vi "Manual splitting analysis.vi"() -> ()   [LabVIEW 2013]
uses:
  <vilib>/Math Plots/2D Math Plots/2D Error Bar/2D Error Bar XCtrl/2D Error Bar.xctl
  <vilib>/Math Plots/2D Math Plots/2D Error Bar/2D Error Bar Datatype/2D Error Bar Datatype.lvclass
  <vilib>/Math Plots/2D Math Plots/2D Error Bar/2D Error Bar Datatype/Public/Plot Helper (Percentage).vi
  <vilib>/Analysis/NI_AALPro.lvlib
panel:
  out "Tab Control":enum32{"Page 1", "Page 2", "ITX"}(tab)=enum."ITX"
  in  "OK Button":bool
  in  "Peak Detector":cluster{"X":dbl, "Y":dbl}[](graph)=[{"X"=-0.049280000000000004, "Y"=-90000.0}, {"X"=-0.04744, "Y"=-90000.0}, {"X"=-0.044360000000000004, "Y"=-90000.0}, {"X"=-0.04356, "Y"=-90000.0}, {"X"=-0.04252, "Y"=-90000.0}, {"X"=-0.0412, "Y"=-90000.0}, {"X"=-0.040080000000000005, "Y"=-90000.0}, {"X"=-0.038000000000000006, "Y"=-90000.0}, {"X"=-0.0374, "Y"=-90000.0}, {"X"=-0.03572, "Y"=-90000.0}, {"X"=-0.035160000000000004, "Y"=-90000.0}, {"X"=-0.032920000000000005, "Y"=-90000.0}, {"X"=-0.03064, "Y"=-90000.0}, {"X"=-0.02964, "Y"=-90000.0}, {"X"=-0.02828, "Y"=-90000.0}, {"X"=-0.02604, "Y"=-90000.0}, {"X"=-0.0246, "Y"=-90000.0}, {"X"=-0.02304, "Y"=-90000.0}, {"X"=-0.022000000000000002, "Y"=-90000.0}, {"X"=-0.02084, "Y"=-90000.0}, {"X"=-0.02, "Y"=-90000.0}, {"X"=-0.017, "Y"=-90000.0}, {"X"=-0.014600000000000002, "Y"=-90000.0}, {"X"=-0.0138, "Y"=-90000.0}, {"X"=-0.013240000000000002, "Y"=-90000.0}, {"X"=-0.011999999999999997, "Y"=-90000.0}, {"X"=-0.01088, "Y"=-90000.0}, {"X"=-0.0102, "Y"=-90000.0}, {"X"=-0.009759999999999998, "Y"=-90000.0}, {"X"=-0.00884, "Y"=-90000.0}, {"X"=-0.007120000000000001, "Y"=-90000.0}, {"X"=-0.0056799999999999976, "Y"=-90000.0}, {"X"=-0.00476, "Y"=-90000.0}, {"X"=-0.049280000000000004, "Y"=-87906.98}, {"X"=-0.04812, "Y"=-87906.98}, {"X"=-0.04624, "Y"=-87906.98}, {"X"=-0.04496, "Y"=-87906.98}, {"X"=-0.04428, "Y"=-87906.98}, {"X"=-0.043000000000000003, "Y"=-87906.98}, {"X"=-0.04184, "Y"=-87906.98}, {"X"=-0.040720000000000006, "Y"=-87906.98}, {"X"=-0.03852, "Y"=-87906.98}, {"X"=-0.037880000000000004, "Y"=-87906.98}, {"X"=-0.03608, "Y"=-87906.98}, {"X"=-0.03556, "Y"=-87906.98}, {"X"=-0.03312, "Y"=-87906.98}, {"X"=-0.031, "Y"=-87906.98}, {"X"=-0.02976, "Y"=-87906.98}, {"X"=-0.028560000000000002, "Y"=-87906.98}, {"X"=-0.02616, "Y"=-87906.98}, {"X"=-0.0248, "Y"=-87906.98}, {"X"=-0.02304, "Y"=-87906.98}, {"X"=-0.02228, "Y"=-87906.98}, {"X"=-0.02172, "Y"=-87906.98}, {"X"=-0.021, "Y"=-87906.98}, {"X"=-0.019880000000000002, "Y"=-87906.98}, {"X"=-0.016919999999999998, "Y"=-87906.98}, {"X"=-0.015559999999999997, "Y"=-87906.98}, {"X"=-0.01412, "Y"=-87906.98}, {"X"=-0.01312, "Y"=-87906.98}, {"X"=-0.011880000000000002, "Y"=-87906.98}, {"X"=-0.01056, "Y"=-87906.98}, {"X"=-0.009320000000000002, "Y"=-87906.98}, {"X"=-0.0068000000000000005, "Y"=-87906.98}, {"X"=-0.0049999999999999975, "Y"=-87906.98}, {"X"=-0.004519999999999996, "Y"=-87906.98}, {"X"=-0.04828, "Y"=-85813.96}, {"X"=-0.045040000000000004, "Y"=-85813.96}, {"X"=-0.04444, "Y"=-85813.96}, {"X"=-0.042960000000000005, "Y"=-85813.96}, {"X"=-0.041960000000000004, "Y"=-85813.96}, {"X"=-0.04084, "Y"=-85813.96}, {"X"=-0.038560000000000004, "Y"=-85813.96}, {"X"=-0.03728, "Y"=-85813.96}, {"X"=-0.036320000000000005, "Y"=-85813.96}, {"X"=-0.0358, "Y"=-85813.96}, {"X"=-0.033, "Y"=-85813.96}, {"X"=-0.031, "Y"=-85813.96}, {"X"=-0.02956, "Y"=-85813.96}, {"X"=-0.02816, "Y"=-85813.96}, {"X"=-0.02688, "Y"=-85813.96}, {"X"=-0.026000000000000002, "Y"=-85813.96}, {"X"=-0.02468, "Y"=-85813.96}, {"X"=-0.0228, "Y"=-85813.96}, {"X"=-0.02228, "Y"=-85813.96}, {"X"=-0.02084, "Y"=-85813.96}, {"X"=-0.01952, "Y"=-85813.96}, {"X"=-0.016919999999999998, "Y"=-85813.96}, {"X"=-0.013879999999999997, "Y"=-85813.96}, {"X"=-0.012799999999999999, "Y"=-85813.96}, {"X"=-0.011319999999999997, "Y"=-85813.96}, {"X"=-0.0102, "Y"=-85813.96}, {"X"=-0.008879999999999999, "Y"=-85813.96}, {"X"=-0.008, "Y"=-85813.96}, {"X"=-0.006519999999999998, "Y"=-85813.96}, {"X"=-0.04836, "Y"=-83720.94}, {"X"=-0.04508, "Y"=-83720.94}, {"X"=-0.04456, "Y"=-83720.94}, {"X"=-0.043120000000000006, "Y"=-83720.94}, {"X"=-0.04192, "Y"=-83720.94}, {"X"=-0.04088, "Y"=-83720.94}, {"X"=-0.038680000000000006, "Y"=-83720.94}, {"X"=-0.03676, "Y"=-83720.94}, {"X"=-0.03612, "Y"=-83720.94}, {"X"=-0.03572, "Y"=-83720.94}, {"X"=-0.032920000000000005, "Y"=-83720.94}, {"X"=-0.031, "Y"=-83720.94}, {"X"=-0.02936, "Y"=-83720.94}, {"X"=-0.027800000000000002, "Y"=-83720.94}, {"X"=-0.02688, "Y"=-83720.94}, {"X"=-0.025840000000000002, "Y"=-83720.94}, {"X"=-0.02476, "Y"=-83720.94}, {"X"=-0.02284, "Y"=-83720.94}, {"X"=-0.02188, "Y"=-83720.94}, {"X"=-0.02076, "Y"=-83720.94}, {"X"=-0.01928, "Y"=-83720.94}, {"X"=-0.016919999999999998, "Y"=-83720.94}, {"X"=-0.01604, "Y"=-83720.94}, {"X"=-0.014559999999999997, "Y"=-83720.94}, {"X"=-0.013560000000000003, "Y"=-83720.94}, {"X"=-0.012839999999999997, "Y"=-83720.94}, {"X"=-0.012360000000000003, "Y"=-83720.94}, {"X"=-0.010079999999999999, "Y"=-83720.94}, {"X"=-0.008719999999999999, "Y"=-83720.94}, {"X"=-0.005999999999999998, "Y"=-83720.94}, {"X"=-0.005319999999999998, "Y"=-83720.94}, {"X"=-0.048400000000000006, "Y"=-81627.92}, {"X"=-0.045160000000000006, "Y"=-81627.92}, {"X"=-0.044680000000000004, "Y"=-81627.92}, {"X"=-0.043160000000000004, "Y"=-81627.92}, {"X"=-0.042, "Y"=-81627.92}, {"X"=-0.04084, "Y"=-81627.92}, {"X"=-0.03876, "Y"=-81627.92}, {"X"=-0.03676, "Y"=-81627.92}, {"X"=-0.036320000000000005, "Y"=-81627.92}, {"X"=-0.03572, "Y"=-81627.92}, {"X"=-0.032880000000000006, "Y"=-81627.92}, {"X"=-0.03108, "Y"=-81627.92}, {"X"=-0.029400000000000003, "Y"=-81627.92}, {"X"=-0.028800000000000003, "Y"=-81627.92}, {"X"=-0.02688, "Y"=-81627.92}, {"X"=-0.02576, "Y"=-81627.92}, {"X"=-0.0248, "Y"=-81627.92}, {"X"=-0.0228, "Y"=-81627.92}, {"X"=-0.02228, "Y"=-81627.92}, {"X"=-0.0216, "Y"=-81627.92}, {"X"=-0.0208, "Y"=-81627.92}, {"X"=-0.019200000000000002, "Y"=-81627.92}, {"X"=-0.016919999999999998, "Y"=-81627.92}, {"X"=-0.01584, "Y"=-81627.92}, {"X"=-0.01328, "Y"=-81627.92}, {"X"=-0.012799999999999999, "Y"=-81627.92}, {"X"=-0.010119999999999997, "Y"=-81627.92}, {"X"=-0.00884, "Y"=-81627.92}, {"X"=-0.00816, "Y"=-81627.92}, {"X"=-0.007919999999999996, "Y"=-81627.92}, {"X"=-0.005999999999999998, "Y"=-81627.92}, {"X"=-0.005719999999999996, "Y"=-81627.92}, {"X"=-0.04848, "Y"=-79534.9}, {"X"=-0.04524, "Y"=-79534.9}, {"X"=-0.04472, "Y"=-79534.9}, {"X"=-0.04308, "Y"=-79534.9}, {"X"=-0.04204, "Y"=-79534.9}, {"X"=-0.041080000000000005, "Y"=-79534.9}, {"X"=-0.03884, "Y"=-79534.9}, {"X"=-0.03696, "Y"=-79534.9}, {"X"=-0.03588, "Y"=-79534.9}, {"X"=-0.032880000000000006, "Y"=-79534.9}, {"X"=-0.031200000000000002, "Y"=-79534.9}, {"X"=-0.029240000000000002, "Y"=-79534.9}, {"X"=-0.028640000000000002, "Y"=-79534.9}, {"X"=-0.02704, "Y"=-79534.9}, {"X"=-0.02572, "Y"=-79534.9}, {"X"=-0.02496, "Y"=-79534.9}, {"X"=-0.0216, "Y"=-79534.9}, {"X"=-0.02088, "Y"=-79534.9}, {"X"=-0.01908, "Y"=-79534.9}, {"X"=-0.01688, "Y"=-79534.9}, {"X"=-0.015600000000000003, "Y"=-79534.9}, {"X"=-0.013479999999999999, "Y"=-79534.9}, {"X"=-0.012720000000000002, "Y"=-79534.9}, {"X"=-0.010000000000000002, "Y"=-79534.9}, {"X"=-0.009000000000000001, "Y"=-79534.9}, {"X"=-0.007679999999999999, "Y"=-79534.9}, {"X"=-0.0058, "Y"=-79534.9}, {"X"=-0.005359999999999997, "Y"=-79534.9}, {"X"=-0.004720000000000002, "Y"=-79534.9}, {"X"=-0.048400000000000006, "Y"=-77441.88}, {"X"=-0.04524, "Y"=-77441.88}, {"X"=-0.04464, "Y"=-77441.88}, {"X"=-0.04292, "Y"=-77441.88}, {"X"=-0.04204, "Y"=-77441.88}, {"X"=-0.04132, "Y"=-77441.88}, {"X"=-0.040760000000000005, "Y"=-77441.88}, {"X"=-0.03888, "Y"=-77441.88}, {"X"=-0.0376, "Y"=-77441.88}, {"X"=-0.03684, "Y"=-77441.88}, {"X"=-0.0358, "Y"=-77441.88}, {"X"=-0.03276, "Y"=-77441.88}, {"X"=-0.03124, "Y"=-77441.88}, {"X"=-0.02908, "Y"=-77441.88}, {"X"=-0.02776, "Y"=-77441.88}, {"X"=-0.02696, "Y"=-77441.88}, {"X"=-0.02496, "Y"=-77441.88}, {"X"=-0.02228, "Y"=-77441.88}, {"X"=-0.02156, "Y"=-77441.88}, {"X"=-0.0208, "Y"=-77441.88}, {"X"=-0.01892, "Y"=-77441.88}, {"X"=-0.01684, "Y"=-77441.88}, {"X"=-0.015280000000000002, "Y"=-77441.88}, {"X"=-0.013319999999999999, "Y"=-77441.88}, {"X"=-0.012519999999999996, "Y"=-77441.88}, {"X"=-0.009840000000000002, "Y"=-77441.88}, {"X"=-0.00884, "Y"=-77441.88}, {"X"=-0.007759999999999996, "Y"=-77441.88}, {"X"=-0.00528, "Y"=-77441.88}, {"X"=-0.04836, "Y"=-75348.86}, {"X"=-0.045200000000000004, "Y"=-75348.86}, {"X"=-0.04456, "Y"=-75348.86}, {"X"=-0.04204, "Y"=-75348.86}, {"X"=-0.041440000000000005, "Y"=-75348.86}, {"X"=-0.040720000000000006, "Y"=-75348.86}, {"X"=-0.0388, "Y"=-75348.86}, {"X"=-0.0374, "Y"=-75348.86}, {"X"=-0.03696, "Y"=-75348.86}, {"X"=-0.03656, "Y"=-75348.86}, {"X"=-0.03572, "Y"=-75348.86}, {"X"=-0.032600000000000004, "Y"=-75348.86}, {"X"=-0.03116, "Y"=-75348.86}, {"X"=-0.02896, "Y"=-75348.86}, {"X"=-0.0276, "Y"=-75348.86}, {"X"=-0.02696, "Y"=-75348.86}, {"X"=-0.02496, "Y"=-75348.86}, {"X"=-0.02152, "Y"=-75348.86}, {"X"=-0.02112, "Y"=-75348.86}, {"X"=-0.0206, "Y"=-75348.86}, {"X"=-0.0188, "Y"=-75348.86}, {"X"=-0.016759999999999997, "Y"=-75348.86}, {"X"=-0.015239999999999997, "Y"=-75348.86}, {"X"=-0.013400000000000002, "Y"=-75348.86}, {"X"=-0.012560000000000002, "Y"=-75348.86}, {"X"=-0.00988, "Y"=-75348.86}, {"X"=-0.008800000000000002, "Y"=-75348.86}, {"X"=-0.00732, "Y"=-75348.86}, {"X"=-0.005359999999999997, "Y"=-75348.86}, {"X"=-0.004799999999999999, "Y"=-75348.86}, {"X"=-0.04836, "Y"=-73255.84}, {"X"=-0.04528, "Y"=-73255.84}, {"X"=-0.044520000000000004, "Y"=-73255.84}, {"X"=-0.04216, "Y"=-73255.84}, {"X"=-0.04148, "Y"=-73255.84}, {"X"=-0.04068, "Y"=-73255.84}, {"X"=-0.0388, "Y"=-73255.84}, {"X"=-0.037680000000000005, "Y"=-73255.84}, {"X"=-0.03716, "Y"=-73255.84}, {"X"=-0.036680000000000004, "Y"=-73255.84}, {"X"=-0.03572, "Y"=-73255.84}, {"X"=-0.033560000000000006, "Y"=-73255.84}, {"X"=-0.032600000000000004, "Y"=-73255.84}, {"X"=-0.03124, "Y"=-73255.84}, {"X"=-0.02888, "Y"=-73255.84}, {"X"=-0.02816, "Y"=-73255.84}, {"X"=-0.02708, "Y"=-73255.84}, {"X"=-0.02504, "Y"=-73255.84}, {"X"=-0.02136, "Y"=-73255.84}, {"X"=-0.02084, "Y"=-73255.84}, {"X"=-0.018520000000000002, "Y"=-73255.84}, {"X"=-0.01672, "Y"=-73255.84}, {"X"=-0.015120000000000001, "Y"=-73255.84}, {"X"=-0.013159999999999998, "Y"=-73255.84}, {"X"=-0.01228, "Y"=-73255.84}, {"X"=-0.01004, "Y"=-73255.84}, {"X"=-0.009119999999999996, "Y"=-73255.84}, {"X"=-0.008800000000000002, "Y"=-73255.84}, {"X"=-0.0074800000000000005, "Y"=-73255.84}, {"X"=-0.005719999999999996, "Y"=-73255.84}, {"X"=-0.00528, "Y"=-73255.84}, {"X"=-0.004720000000000002, "Y"=-73255.84}, {"X"=-0.0478, "Y"=-71162.82}, {"X"=-0.04532, "Y"=-71162.82}, {"X"=-0.044320000000000005, "Y"=-71162.82}, {"X"=-0.04184, "Y"=-71162.82}, {"X"=-0.04124, "Y"=-71162.82}, {"X"=-0.040440000000000004, "Y"=-71162.82}, {"X"=-0.039240000000000004, "Y"=-71162.82}, {"X"=-0.03852, "Y"=-71162.82}, {"X"=-0.03724, "Y"=-71162.82}, {"X"=-0.0366, "Y"=-71162.82}, {"X"=-0.03536, "Y"=-71162.82}, {"X"=-0.034, "Y"=-71162.82}, {"X"=-0.032200000000000006, "Y"=-71162.82}, {"X"=-0.03092, "Y"=-71162.82}, {"X"=-0.028800000000000003, "Y"=-71162.82}, {"X"=-0.02688, "Y"=-71162.82}, {"X"=-0.025, "Y"=-71162.82}, {"X"=-0.02112, "Y"=-71162.82}, {"X"=-0.02068, "Y"=-71162.82}, {"X"=-0.018439999999999998, "Y"=-71162.82}, {"X"=-0.01636, "Y"=-71162.82}, {"X"=-0.014839999999999999, "Y"=-71162.82}, {"X"=-0.01328, "Y"=-71162.82}, {"X"=-0.012880000000000003, "Y"=-71162.82}, {"X"=-0.01228, "Y"=-71162.82}, {"X"=-0.009640000000000003, "Y"=-71162.82}, {"X"=-0.009160000000000001, "Y"=-71162.82}, {"X"=-0.007280000000000002, "Y"=-71162.82}, {"X"=-0.0051199999999999996, "Y"=-71162.82}, {"X"=-0.048, "Y"=-69069.8}, {"X"=-0.04564, "Y"=-69069.8}, {"X"=-0.044480000000000006, "Y"=-69069.8}, {"X"=-0.04224, "Y"=-69069.8}, {"X"=-0.04152, "Y"=-69069.8}, {"X"=-0.04068, "Y"=-69069.8}, {"X"=-0.03948, "Y"=-69069.8}, {"X"=-0.03884, "Y"=-69069.8}, {"X"=-0.03828, "Y"=-69069.8}, {"X"=-0.03776, "Y"=-69069.8}, {"X"=-0.03692, "Y"=-69069.8}, {"X"=-0.03552, "Y"=-69069.8}, {"X"=-0.03416, "Y"=-69069.8}, {"X"=-0.0324, "Y"=-69069.8}, {"X"=-0.03104, "Y"=-69069.8}, {"X"=-0.02896, "Y"=-69069.8}, {"X"=-0.02716, "Y"=-69069.8}, {"X"=-0.025240000000000002, "Y"=-69069.8}, {"X"=-0.024560000000000002, "Y"=-69069.8}, {"X"=-0.02104, "Y"=-69069.8}, {"X"=-0.02024, "Y"=-69069.8}, {"X"=-0.01824, "Y"=-69069.8}, {"X"=-0.01652, "Y"=-69069.8}, {"X"=-0.014559999999999997, "Y"=-69069.8}, {"X"=-0.01328, "Y"=-69069.8}, {"X"=-0.011999999999999997, "Y"=-69069.8}, {"X"=-0.009559999999999999, "Y"=-69069.8}, {"X"=-0.00884, "Y"=-69069.8}, {"X"=-0.0072399999999999964, "Y"=-69069.8}, {"X"=-0.00544, "Y"=-69069.8}, {"X"=-0.04812, "Y"=-66976.78}, {"X"=-0.045360000000000004, "Y"=-66976.78}, {"X"=-0.044320000000000005, "Y"=-66976.78}, {"X"=-0.04156, "Y"=-66976.78}, {"X"=-0.04056, "Y"=-66976.78}, {"X"=-0.03884, "Y"=-66976.78}, {"X"=-0.03764, "Y"=-66976.78}, {"X"=-0.03684, "Y"=-66976.78}, {"X"=-0.03548, "Y"=-66976.78}, {"X"=-0.03344, "Y"=-66976.78}, {"X"=-0.0324, "Y"=-66976.78}, {"X"=-0.03148, "Y"=-66976.78}, {"X"=-0.0302, "Y"=-66976.78}, {"X"=-0.028720000000000002, "Y"=-66976.78}, {"X"=-0.02704, "Y"=-66976.78}, {"X"=-0.02508, "Y"=-66976.78}, {"X"=-0.021320000000000002, "Y"=-66976.78}, {"X"=-0.02048, "Y"=-66976.78}, {"X"=-0.01836, "Y"=-66976.78}, {"X"=-0.016800000000000002, "Y"=-66976.78}, {"X"=-0.015559999999999997, "Y"=-66976.78}, {"X"=-0.014600000000000002, "Y"=-66976.78}, {"X"=-0.013519999999999997, "Y"=-66976.78}, {"X"=-0.012360000000000003, "Y"=-66976.78}, {"X"=-0.010119999999999997, "Y"=-66976.78}, {"X"=-0.009160000000000001, "Y"=-66976.78}, {"X"=-0.007519999999999999, "Y"=-66976.78}, {"X"=-0.006280000000000001, "Y"=-66976.78}, {"X"=-0.005240000000000002, "Y"=-66976.78}, {"X"=-0.0482, "Y"=-64883.76}, {"X"=-0.045520000000000005, "Y"=-64883.76}, {"X"=-0.044360000000000004, "Y"=-64883.76}, {"X"=-0.04192, "Y"=-64883.76}, {"X"=-0.04056, "Y"=-64883.76}, {"X"=-0.03896, "Y"=-64883.76}, {"X"=-0.03808, "Y"=-64883.76}, {"X"=-0.037720000000000004, "Y"=-64883.76}, {"X"=-0.03696, "Y"=-64883.76}, {"X"=-0.03544, "Y"=-64883.76}, {"X"=-0.03352, "Y"=-64883.76}, {"X"=-0.0324, "Y"=-64883.76}, {"X"=-0.0316, "Y"=-64883.76}, {"X"=-0.03036, "Y"=-64883.76}, {"X"=-0.028720000000000002, "Y"=-64883.76}, {"X"=-0.027, "Y"=-64883.76}, {"X"=-0.025160000000000002, "Y"=-64883.76}, {"X"=-0.02148, "Y"=-64883.76}, {"X"=-0.02036, "Y"=-64883.76}, {"X"=-0.01824, "Y"=-64883.76}, {"X"=-0.01684, "Y"=-64883.76}, {"X"=-0.01568, "Y"=-64883.76}, {"X"=-0.014359999999999998, "Y"=-64883.76}, {"X"=-0.013679999999999998, "Y"=-64883.76}, {"X"=-0.012200000000000003, "Y"=-64883.76}, {"X"=-0.009399999999999999, "Y"=-64883.76}, {"X"=-0.0072399999999999964, "Y"=-64883.76}, {"X"=-0.006399999999999996, "Y"=-64883.76}, {"X"=-0.04804, "Y"=-62790.740000000005}, {"X"=-0.04548, "Y"=-62790.740000000005}, {"X"=-0.04424, "Y"=-62790.740000000005}, {"X"=-0.04192, "Y"=-62790.740000000005}, {"X"=-0.04124, "Y"=-62790.740000000005}, {"X"=-0.040440000000000004, "Y"=-62790.740000000005}, {"X"=-0.03892, "Y"=-62790.740000000005}, {"X"=-0.03792, "Y"=-62790.740000000005}, {"X"=-0.03692, "Y"=-62790.740000000005}, {"X"=-0.035320000000000004, "Y"=-62790.740000000005}, {"X"=-0.03344, "Y"=-62790.740000000005}, {"X"=-0.03228, "Y"=-62790.740000000005}, {"X"=-0.0316, "Y"=-62790.740000000005}, {"X"=-0.0304, "Y"=-62790.740000000005}, {"X"=-0.028640000000000002, "Y"=-62790.740000000005}, {"X"=-0.02696, "Y"=-62790.740000000005}, {"X"=-0.025240000000000002, "Y"=-62790.740000000005}, {"X"=-0.02148, "Y"=-62790.740000000005}, {"X"=-0.02016, "Y"=-62790.740000000005}, {"X"=-0.0182, "Y"=-62790.740000000005}, {"X"=-0.016960000000000003, "Y"=-62790.740000000005}, {"X"=-0.015719999999999998, "Y"=-62790.740000000005}, {"X"=-0.01412, "Y"=-62790.740000000005}, {"X"=-0.013760000000000001, "Y"=-62790.740000000005}, {"X"=-0.01228, "Y"=-62790.740000000005}, {"X"=-0.011680000000000003, "Y"=-62790.740000000005}, {"X"=-0.009559999999999999, "Y"=-62790.740000000005}, {"X"=-0.00732, "Y"=-62790.740000000005}, {"X"=-0.0062400000000000025, "Y"=-62790.740000000005}, {"X"=-0.005639999999999999, "Y"=-62790.740000000005}, {"X"=-0.048, "Y"=-60697.72}, {"X"=-0.04556, "Y"=-60697.72}, {"X"=-0.044160000000000005, "Y"=-60697.72}, {"X"=-0.04192, "Y"=-60697.72}, {"X"=-0.041120000000000004, "Y"=-60697.72}, {"X"=-0.04028, "Y"=-60697.72}, {"X"=-0.039080000000000004, "Y"=-60697.72}, {"X"=-0.0386, "Y"=-60697.72}, {"X"=-0.03792, "Y"=-60697.72}, {"X"=-0.03696, "Y"=-60697.72}, {"X"=-0.03524, "Y"=-60697.72}, {"X"=-0.0334, "Y"=-60697.72}, {"X"=-0.03204, "Y"=-60697.72}, {"X"=-0.03184, "Y"=-60697.72}, {"X"=-0.03048, "Y"=-60697.72}, {"X"=-0.028560000000000002, "Y"=-60697.72}, {"X"=-0.02764, "Y"=-60697.72}, {"X"=-0.02528, "Y"=-60697.72}, {"X"=-0.02148, "Y"=-60697.72}, {"X"=-0.02, "Y"=-60697.72}, {"X"=-0.018160000000000003, "Y"=-60697.72}, {"X"=-0.015919999999999997, "Y"=-60697.72}, {"X"=-0.013879999999999997, "Y"=-60697.72}, {"X"=-0.012240000000000001, "Y"=-60697.72}, {"X"=-0.009680000000000001, "Y"=-60697.72}, {"X"=-0.007440000000000002, "Y"=-60697.72}, {"X"=-0.006359999999999998, "Y"=-60697.72}, {"X"=-0.0058, "Y"=-60697.72}, {"X"=-0.00528, "Y"=-60697.72}, {"X"=-0.047920000000000004, "Y"=-58604.7}, {"X"=-0.04556, "Y"=-58604.7}, {"X"=-0.044000000000000004, "Y"=-58604.7}, {"X"=-0.04192, "Y"=-58604.7}, {"X"=-0.041080000000000005, "Y"=-58604.7}, {"X"=-0.04016, "Y"=-58604.7}, {"X"=-0.039040000000000005, "Y"=-58604.7}, {"X"=-0.03808, "Y"=-58604.7}, {"X"=-0.03692, "Y"=-58604.7}, {"X"=-0.035160000000000004, "Y"=-58604.7}, {"X"=-0.0334, "Y"=-58604.7}, {"X"=-0.031920000000000004, "Y"=-58604.7}, {"X"=-0.030520000000000002, "Y"=-58604.7}, {"X"=-0.028480000000000002, "Y"=-58604.7}, {"X"=-0.027440000000000003, "Y"=-58604.7}, {"X"=-0.025400000000000002, "Y"=-58604.7}, {"X"=-0.02476, "Y"=-58604.7}, {"X"=-0.0216, "Y"=-58604.7}, {"X"=-0.02, "Y"=-58604.7}, {"X"=-0.018119999999999997, "Y"=-58604.7}, {"X"=-0.016399999999999998, "Y"=-58604.7}, {"X"=-0.013999999999999999, "Y"=-58604.7}, {"X"=-0.01228, "Y"=-58604.7}, {"X"=-0.009799999999999996, "Y"=-58604.7}, {"X"=-0.007519999999999999, "Y"=-58604.7}, {"X"=-0.0068000000000000005, "Y"=-58604.7}, {"X"=-0.0061200000000000004, "Y"=-58604.7}, {"X"=-0.0049999999999999975, "Y"=-58604.7}, {"X"=-0.004519999999999996, "Y"=-58604.7}, {"X"=-0.04832, "Y"=-56511.68}, {"X"=-0.04624, "Y"=-56511.68}, {"X"=-0.04424, "Y"=-56511.68}, {"X"=-0.04232, "Y"=-56511.68}, {"X"=-0.04136, "Y"=-56511.68}, {"X"=-0.04028, "Y"=-56511.68}, {"X"=-0.03952, "Y"=-56511.68}, {"X"=-0.03896, "Y"=-56511.68}, {"X"=-0.03824, "Y"=-56511.68}, {"X"=-0.03728, "Y"=-56511.68}, {"X"=-0.03524, "Y"=-56511.68}, {"X"=-0.0342, "Y"=-56511.68}, {"X"=-0.03316, "Y"=-56511.68}, {"X"=-0.03184, "Y"=-56511.68}, {"X"=-0.03056, "Y"=-56511.68}, {"X"=-0.028480000000000002, "Y"=-56511.68}, {"X"=-0.028, "Y"=-56511.68}, {"X"=-0.02544, "Y"=-56511.68}, {"X"=-0.024640000000000002, "Y"=-56511.68}, {"X"=-0.02164, "Y"=-56511.68}, {"X"=-0.02004, "Y"=-56511.68}, {"X"=-0.01804, "Y"=-56511.68}, {"X"=-0.01636, "Y"=-56511.68}, {"X"=-0.013999999999999999, "Y"=-56511.68}, {"X"=-0.011959999999999998, "Y"=-56511.68}, {"X"=-0.00988, "Y"=-56511.68}, {"X"=-0.0072399999999999964, "Y"=-56511.68}, {"X"=-0.0068000000000000005, "Y"=-56511.68}, {"X"=-0.004920000000000001, "Y"=-56511.68}, {"X"=-0.048240000000000005, "Y"=-54418.66}, {"X"=-0.04624, "Y"=-54418.66}, {"X"=-0.04404, "Y"=-54418.66}, {"X"=-0.042280000000000005, "Y"=-54418.66}, {"X"=-0.041, "Y"=-54418.66}, {"X"=-0.04028, "Y"=-54418.66}, {"X"=-0.039400000000000004, "Y"=-54418.66}, {"X"=-0.039, "Y"=-54418.66}, {"X"=-0.0382, "Y"=-54418.66}, {"X"=-0.03728, "Y"=-54418.66}, {"X"=-0.035160000000000004, "Y"=-54418.66}, {"X"=-0.03416, "Y"=-54418.66}, {"X"=-0.03212, "Y"=-54418.66}, {"X"=-0.030160000000000003, "Y"=-54418.66}, {"X"=-0.02816, "Y"=-54418.66}, {"X"=-0.02748, "Y"=-54418.66}, {"X"=-0.02548, "Y"=-54418.66}, {"X"=-0.024560000000000002, "Y"=-54418.66}, {"X"=-0.02176, "Y"=-54418.66}, {"X"=-0.01992, "Y"=-54418.66}, {"X"=-0.018000000000000002, "Y"=-54418.66}, {"X"=-0.017320000000000002, "Y"=-54418.66}, {"X"=-0.016399999999999998, "Y"=-54418.66}, {"X"=-0.01412, "Y"=-54418.66}, {"X"=-0.011880000000000002, "Y"=-54418.66}, {"X"=-0.009919999999999998, "Y"=-54418.66}, {"X"=-0.0074800000000000005, "Y"=-54418.66}, {"X"=-0.006159999999999999, "Y"=-54418.66}, {"X"=-0.004720000000000002, "Y"=-54418.66}, {"X"=-0.04812, "Y"=-52325.64}, {"X"=-0.04624, "Y"=-52325.64}, {"X"=-0.04396, "Y"=-52325.64}, {"X"=-0.042280000000000005, "Y"=-52325.64}, {"X"=-0.0412, "Y"=-52325.64}, {"X"=-0.040600000000000004, "Y"=-52325.64}, {"X"=-0.03996, "Y"=-52325.64}, {"X"=-0.03932, "Y"=-52325.64}, {"X"=-0.03916, "Y"=-52325.64}, {"X"=-0.0382, "Y"=-52325.64}, {"X"=-0.03684, "Y"=-52325.64}, {"X"=-0.03492, "Y"=-52325.64}, {"X"=-0.0332, "Y"=-52325.64}, {"X"=-0.03176, "Y"=-52325.64}, {"X"=-0.03072, "Y"=-52325.64}, {"X"=-0.02784, "Y"=-52325.64}, {"X"=-0.02556, "Y"=-52325.64}, {"X"=-0.024480000000000002, "Y"=-52325.64}, {"X"=-0.021840000000000002, "Y"=-52325.64}, {"X"=-0.02076, "Y"=-52325.64}, {"X"=-0.01976, "Y"=-52325.64}, {"X"=-0.01804, "Y"=-52325.64}, {"X"=-0.016399999999999998, "Y"=-52325.64}, {"X"=-0.015960000000000002, "Y"=-52325.64}, {"X"=-0.014240000000000003, "Y"=-52325.64}, {"X"=-0.011880000000000002, "Y"=-52325.64}, {"X"=-0.010119999999999997, "Y"=-52325.64}, {"X"=-0.0072399999999999964, "Y"=-52325.64}, {"X"=-0.006600000000000002, "Y"=-52325.64}, {"X"=-0.0049999999999999975, "Y"=-52325.64}, {"X"=-0.04804, "Y"=-50232.62}, {"X"=-0.04624, "Y"=-50232.62}, {"X"=-0.043840000000000004, "Y"=-50232.62}, {"X"=-0.04224, "Y"=-50232.62}, {"X"=-0.04104, "Y"=-50232.62}, {"X"=-0.040080000000000005, "Y"=-50232.62}, {"X"=-0.039040000000000005, "Y"=-50232.62}, {"X"=-0.03808, "Y"=-50232.62}, {"X"=-0.037320000000000006, "Y"=-50232.62}, {"X"=-0.035, "Y"=-50232.62}, {"X"=-0.034, "Y"=-50232.62}, {"X"=-0.03212, "Y"=-50232.62}, {"X"=-0.03144, "Y"=-50232.62}, {"X"=-0.02904, "Y"=-50232.62}, {"X"=-0.02776, "Y"=-50232.62}, {"X"=-0.02556, "Y"=-50232.62}, {"X"=-0.02432, "Y"=-50232.62}, {"X"=-0.021840000000000002, "Y"=-50232.62}, {"X"=-0.01984, "Y"=-50232.62}, {"X"=-0.01792, "Y"=-50232.62}, {"X"=-0.014280000000000001, "Y"=-50232.62}, {"X"=-0.011680000000000003, "Y"=-50232.62}, {"X"=-0.010079999999999999, "Y"=-50232.62}, {"X"=-0.00732, "Y"=-50232.62}, {"X"=-0.00648, "Y"=-50232.62}, {"X"=-0.0055600000000000024, "Y"=-50232.62}, {"X"=-0.004959999999999999, "Y"=-50232.62}, {"X"=-0.04796, "Y"=-48139.6}, {"X"=-0.04628, "Y"=-48139.6}, {"X"=-0.04376, "Y"=-48139.6}, {"X"=-0.042280000000000005, "Y"=-48139.6}, {"X"=-0.041, "Y"=-48139.6}, {"X"=-0.04032, "Y"=-48139.6}, {"X"=-0.03896, "Y"=-48139.6}, {"X"=-0.038680000000000006, "Y"=-48139.6}, {"X"=-0.038000000000000006, "Y"=-48139.6}, {"X"=-0.03696, "Y"=-48139.6}, {"X"=-0.0348, "Y"=-48139.6}, {"X"=-0.033, "Y"=-48139.6}, {"X"=-0.03204, "Y"=-48139.6}, {"X"=-0.031520000000000006, "Y"=-48139.6}, {"X"=-0.02908, "Y"=-48139.6}, {"X"=-0.027960000000000002, "Y"=-48139.6}, {"X"=-0.027280000000000002, "Y"=-48139.6}, {"X"=-0.02564, "Y"=-48139.6}, {"X"=-0.02428, "Y"=-48139.6}, {"X"=-0.02196, "Y"=-48139.6}, {"X"=-0.02, "Y"=-48139.6}, {"X"=-0.017959999999999997, "Y"=-48139.6}, {"X"=-0.01736, "Y"=-48139.6}, {"X"=-0.01448, "Y"=-48139.6}, {"X"=-0.0116, "Y"=-48139.6}, {"X"=-0.010160000000000002, "Y"=-48139.6}, {"X"=-0.009439999999999997, "Y"=-48139.6}, {"X"=-0.006719999999999997, "Y"=-48139.6}, {"X"=-0.005359999999999997, "Y"=-48139.6}, {"X"=-0.048, "Y"=-46046.58}, {"X"=-0.046400000000000004, "Y"=-46046.58}, {"X"=-0.043800000000000006, "Y"=-46046.58}, {"X"=-0.042440000000000005, "Y"=-46046.58}, {"X"=-0.041960000000000004, "Y"=-46046.58}, {"X"=-0.040720000000000006, "Y"=-46046.58}, {"X"=-0.040440000000000004, "Y"=-46046.58}, {"X"=-0.039360000000000006, "Y"=-46046.58}, {"X"=-0.03876, "Y"=-46046.58}, {"X"=-0.03808, "Y"=-46046.58}, {"X"=-0.03716, "Y"=-46046.58}, {"X"=-0.03484, "Y"=-46046.58}, {"X"=-0.03312, "Y"=-46046.58}, {"X"=-0.03228, "Y"=-46046.58}, {"X"=-0.031560000000000005, "Y"=-46046.58}, {"X"=-0.02928, "Y"=-46046.58}, {"X"=-0.028120000000000003, "Y"=-46046.58}, {"X"=-0.02768, "Y"=-46046.58}, {"X"=-0.025920000000000002, "Y"=-46046.58}, {"X"=-0.02436, "Y"=-46046.58}, {"X"=-0.0222, "Y"=-46046.58}, {"X"=-0.02012, "Y"=-46046.58}, {"X"=-0.01972, "Y"=-46046.58}, {"X"=-0.0182, "Y"=-46046.58}, {"X"=-0.017480000000000002, "Y"=-46046.58}, {"X"=-0.0148, "Y"=-46046.58}, {"X"=-0.01396, "Y"=-46046.58}, {"X"=-0.011839999999999996, "Y"=-46046.58}, {"X"=-0.010599999999999998, "Y"=-46046.58}, {"X"=-0.009680000000000001, "Y"=-46046.58}, {"X"=-0.0069200000000000025, "Y"=-46046.58}, {"X"=-0.006319999999999999, "Y"=-46046.58}, {"X"=-0.0058, "Y"=-46046.58}, {"X"=-0.005359999999999997, "Y"=-46046.58}, {"X"=-0.047880000000000006, "Y"=-43953.56}, {"X"=-0.046400000000000004, "Y"=-43953.56}, {"X"=-0.043680000000000004, "Y"=-43953.56}, {"X"=-0.042440000000000005, "Y"=-43953.56}, {"X"=-0.041800000000000004, "Y"=-43953.56}, {"X"=-0.0408, "Y"=-43953.56}, {"X"=-0.0402, "Y"=-43953.56}, {"X"=-0.039, "Y"=-43953.56}, {"X"=-0.03776, "Y"=-43953.56}, {"X"=-0.037200000000000004, "Y"=-43953.56}, {"X"=-0.03472, "Y"=-43953.56}, {"X"=-0.033, "Y"=-43953.56}, {"X"=-0.03236, "Y"=-43953.56}, {"X"=-0.03144, "Y"=-43953.56}, {"X"=-0.02928, "Y"=-43953.56}, {"X"=-0.02792, "Y"=-43953.56}, {"X"=-0.02596, "Y"=-43953.56}, {"X"=-0.0242, "Y"=-43953.56}, {"X"=-0.02224, "Y"=-43953.56}, {"X"=-0.02008, "Y"=-43953.56}, {"X"=-0.01964, "Y"=-43953.56}, {"X"=-0.018160000000000003, "Y"=-43953.56}, {"X"=-0.01736, "Y"=-43953.56}, {"X"=-0.014879999999999997, "Y"=-43953.56}, {"X"=-0.013760000000000001, "Y"=-43953.56}, {"X"=-0.01176, "Y"=-43953.56}, {"X"=-0.010479999999999996, "Y"=-43953.56}, {"X"=-0.009840000000000002, "Y"=-43953.56}, {"X"=-0.009399999999999999, "Y"=-43953.56}, {"X"=-0.008039999999999999, "Y"=-43953.56}, {"X"=-0.0066799999999999984, "Y"=-43953.56}, {"X"=-0.005359999999999997, "Y"=-43953.56}, {"X"=-0.047200000000000006, "Y"=-41860.54}, {"X"=-0.04576, "Y"=-41860.54}, {"X"=-0.04324, "Y"=-41860.54}, {"X"=-0.042120000000000005, "Y"=-41860.54}, {"X"=-0.04056, "Y"=-41860.54}, {"X"=-0.03984, "Y"=-41860.54}, {"X"=-0.0386, "Y"=-41860.54}, {"X"=-0.038040000000000004, "Y"=-41860.54}, {"X"=-0.03748, "Y"=-41860.54}, {"X"=-0.03456, "Y"=-41860.54}, {"X"=-0.0324, "Y"=-41860.54}, {"X"=-0.03132, "Y"=-41860.54}, {"X"=-0.029240000000000002, "Y"=-41860.54}, {"X"=-0.02784, "Y"=-41860.54}, {"X"=-0.02716, "Y"=-41860.54}, {"X"=-0.02596, "Y"=-41860.54}, {"X"=-0.024, "Y"=-41860.54}, {"X"=-0.02228, "Y"=-41860.54}, {"X"=-0.02004, "Y"=-41860.54}, {"X"=-0.018160000000000003, "Y"=-41860.54}, {"X"=-0.017320000000000002, "Y"=-41860.54}, {"X"=-0.015039999999999998, "Y"=-41860.54}, {"X"=-0.013760000000000001, "Y"=-41860.54}, {"X"=-0.011880000000000002, "Y"=-41860.54}, {"X"=-0.011319999999999997, "Y"=-41860.54}, {"X"=-0.010599999999999998, "Y"=-41860.54}, {"X"=-0.00972, "Y"=-41860.54}, {"X"=-0.007039999999999998, "Y"=-41860.54}, {"X"=-0.005479999999999999, "Y"=-41860.54}, {"X"=-0.00528, "Y"=-41860.54}, {"X"=-0.047080000000000004, "Y"=-39767.520000000004}, {"X"=-0.045720000000000004, "Y"=-39767.520000000004}, {"X"=-0.04308, "Y"=-39767.520000000004}, {"X"=-0.042080000000000006, "Y"=-39767.520000000004}, {"X"=-0.040600000000000004, "Y"=-39767.520000000004}, {"X"=-0.040080000000000005, "Y"=-39767.520000000004}, {"X"=-0.03944, "Y"=-39767.520000000004}, {"X"=-0.03848, "Y"=-39767.520000000004}, {"X"=-0.0378, "Y"=-39767.520000000004}, {"X"=-0.03696, "Y"=-39767.520000000004}, {"X"=-0.03444, "Y"=-39767.520000000004}, {"X"=-0.03244, "Y"=-39767.520000000004}, {"X"=-0.03128, "Y"=-39767.520000000004}, {"X"=-0.029320000000000002, "Y"=-39767.520000000004}, {"X"=-0.02776, "Y"=-39767.520000000004}, {"X"=-0.02664, "Y"=-39767.520000000004}, {"X"=-0.02604, "Y"=-39767.520000000004}, {"X"=-0.023960000000000002, "Y"=-39767.520000000004}, {"X"=-0.02244, "Y"=-39767.520000000004}, {"X"=-0.02028, "Y"=-39767.520000000004}, {"X"=-0.01944, "Y"=-39767.520000000004}, {"X"=-0.018279999999999998, "Y"=-39767.520000000004}, {"X"=-0.017439999999999997, "Y"=-39767.520000000004}, {"X"=-0.015199999999999998, "Y"=-39767.520000000004}, {"X"=-0.013720000000000003, "Y"=-39767.520000000004}, {"X"=-0.011999999999999997, "Y"=-39767.520000000004}, {"X"=-0.01088, "Y"=-39767.520000000004}, {"X"=-0.01004, "Y"=-39767.520000000004}, {"X"=-0.00816, "Y"=-39767.520000000004}, {"X"=-0.006960000000000001, "Y"=-39767.520000000004}, {"X"=-0.005199999999999996, "Y"=-39767.520000000004}, {"X"=-0.004679999999999997, "Y"=-39767.520000000004}, {"X"=-0.04744, "Y"=-37674.5}, {"X"=-0.04628, "Y"=-37674.5}, {"X"=-0.04324, "Y"=-37674.5}, {"X"=-0.0424, "Y"=-37674.5}, {"X"=-0.041440000000000005, "Y"=-37674.5}, {"X"=-0.040720000000000006, "Y"=-37674.5}, {"X"=-0.04016, "Y"=-37674.5}, {"X"=-0.03864, "Y"=-37674.5}, {"X"=-0.037880000000000004, "Y"=-37674.5}, {"X"=-0.0374, "Y"=-37674.5}, {"X"=-0.03432, "Y"=-37674.5}, {"X"=-0.03248, "Y"=-37674.5}, {"X"=-0.03124, "Y"=-37674.5}, {"X"=-0.02928, "Y"=-37674.5}, {"X"=-0.02764, "Y"=-37674.5}, {"X"=-0.02612, "Y"=-37674.5}, {"X"=-0.0238, "Y"=-37674.5}, {"X"=-0.02248, "Y"=-37674.5}, {"X"=-0.02016, "Y"=-37674.5}, {"X"=-0.01928, "Y"=-37674.5}, {"X"=-0.01824, "Y"=-37674.5}, {"X"=-0.01724, "Y"=-37674.5}, {"X"=-0.015280000000000002, "Y"=-37674.5}, {"X"=-0.013519999999999997, "Y"=-37674.5}, {"X"=-0.011479999999999997, "Y"=-37674.5}, {"X"=-0.01092, "Y"=-37674.5}, {"X"=-0.009680000000000001, "Y"=-37674.5}, {"X"=-0.008640000000000002, "Y"=-37674.5}, {"X"=-0.0066799999999999984, "Y"=-37674.5}, {"X"=-0.0051199999999999996, "Y"=-37674.5}, {"X"=-0.04728, "Y"=-35581.48}, {"X"=-0.046200000000000005, "Y"=-35581.48}, {"X"=-0.04308, "Y"=-35581.48}, {"X"=-0.04232, "Y"=-35581.48}, {"X"=-0.04136, "Y"=-35581.48}, {"X"=-0.040760000000000005, "Y"=-35581.48}, {"X"=-0.03848, "Y"=-35581.48}, {"X"=-0.03776, "Y"=-35581.48}, {"X"=-0.03712, "Y"=-35581.48}, {"X"=-0.03416, "Y"=-35581.48}, {"X"=-0.03244, "Y"=-35581.48}, {"X"=-0.03116, "Y"=-35581.48}, {"X"=-0.02936, "Y"=-35581.48}, {"X"=-0.02844, "Y"=-35581.48}, {"X"=-0.02748, "Y"=-35581.48}, {"X"=-0.02612, "Y"=-35581.48}, {"X"=-0.02368, "Y"=-35581.48}, {"X"=-0.02248, "Y"=-35581.48}, {"X"=-0.02008, "Y"=-35581.48}, {"X"=-0.01916, "Y"=-35581.48}, {"X"=-0.018320000000000003, "Y"=-35581.48}, {"X"=-0.017279999999999997, "Y"=-35581.48}, {"X"=-0.015359999999999999, "Y"=-35581.48}, {"X"=-0.01344, "Y"=-35581.48}, {"X"=-0.011839999999999996, "Y"=-35581.48}, {"X"=-0.01092, "Y"=-35581.48}, {"X"=-0.00972, "Y"=-35581.48}, {"X"=-0.006879999999999997, "Y"=-35581.48}, {"X"=-0.004839999999999997, "Y"=-35581.48}, {"X"=-0.047, "Y"=-33488.46}, {"X"=-0.04608, "Y"=-33488.46}, {"X"=-0.04288, "Y"=-33488.46}, {"X"=-0.0422, "Y"=-33488.46}, {"X"=-0.04104, "Y"=-33488.46}, {"X"=-0.04056, "Y"=-33488.46}, {"X"=-0.03988, "Y"=-33488.46}, {"X"=-0.03832, "Y"=-33488.46}, {"X"=-0.0378, "Y"=-33488.46}, {"X"=-0.0342, "Y"=-33488.46}, {"X"=-0.0334, "Y"=-33488.46}, {"X"=-0.03232, "Y"=-33488.46}, {"X"=-0.03096, "Y"=-33488.46}, {"X"=-0.0296, "Y"=-33488.46}, {"X"=-0.02792, "Y"=-33488.46}, {"X"=-0.02664, "Y"=-33488.46}, {"X"=-0.02604, "Y"=-33488.46}, {"X"=-0.02364, "Y"=-33488.46}, {"X"=-0.022520000000000002, "Y"=-33488.46}, {"X"=-0.02, "Y"=-33488.46}, {"X"=-0.01924, "Y"=-33488.46}, {"X"=-0.018320000000000003, "Y"=-33488.46}, {"X"=-0.0172, "Y"=-33488.46}, {"X"=-0.015519999999999999, "Y"=-33488.46}, {"X"=-0.01328, "Y"=-33488.46}, {"X"=-0.0116, "Y"=-33488.46}, {"X"=-0.011200000000000002, "Y"=-33488.46}, {"X"=-0.009799999999999996, "Y"=-33488.46}, {"X"=-0.006839999999999999, "Y"=-33488.46}, {"X"=-0.005240000000000002, "Y"=-33488.46}, {"X"=-0.004839999999999997, "Y"=-33488.46}, {"X"=-0.046520000000000006, "Y"=-31395.440000000002}, {"X"=-0.04564, "Y"=-31395.440000000002}, {"X"=-0.04256, "Y"=-31395.440000000002}, {"X"=-0.042, "Y"=-31395.440000000002}, {"X"=-0.04104, "Y"=-31395.440000000002}, {"X"=-0.03964, "Y"=-31395.440000000002}, {"X"=-0.03912, "Y"=-31395.440000000002}, {"X"=-0.0382, "Y"=-31395.440000000002}, {"X"=-0.037680000000000005, "Y"=-31395.440000000002}, {"X"=-0.037040000000000003, "Y"=-31395.440000000002}, {"X"=-0.03408, "Y"=-31395.440000000002}, {"X"=-0.032560000000000006, "Y"=-31395.440000000002}, {"X"=-0.03136, "Y"=-31395.440000000002}, {"X"=-0.02956, "Y"=-31395.440000000002}, {"X"=-0.02756, "Y"=-31395.440000000002}, {"X"=-0.026600000000000002, "Y"=-31395.440000000002}, {"X"=-0.026080000000000002, "Y"=-31395.440000000002}, {"X"=-0.02368, "Y"=-31395.440000000002}, {"X"=-0.02272, "Y"=-31395.440000000002}, {"X"=-0.02004, "Y"=-31395.440000000002}, {"X"=-0.01968, "Y"=-31395.440000000002}, {"X"=-0.01912, "Y"=-31395.440000000002}, {"X"=-0.018680000000000002, "Y"=-31395.440000000002}, {"X"=-0.017320000000000002, "Y"=-31395.440000000002}, {"X"=-0.015760000000000003, "Y"=-31395.440000000002}, {"X"=-0.013400000000000002, "Y"=-31395.440000000002}, {"X"=-0.011319999999999997, "Y"=-31395.440000000002}, {"X"=-0.010000000000000002, "Y"=-31395.440000000002}, {"X"=-0.0074800000000000005, "Y"=-31395.440000000002}, {"X"=-0.0068000000000000005, "Y"=-31395.440000000002}, {"X"=-0.005719999999999996, "Y"=-31395.440000000002}, {"X"=-0.004799999999999999, "Y"=-31395.440000000002}, {"X"=-0.04644, "Y"=-29302.42}, {"X"=-0.0456, "Y"=-29302.42}, {"X"=-0.042480000000000004, "Y"=-29302.42}, {"X"=-0.04104, "Y"=-29302.42}, {"X"=-0.0398, "Y"=-29302.42}, {"X"=-0.039080000000000004, "Y"=-29302.42}, {"X"=-0.0382, "Y"=-29302.42}, {"X"=-0.037720000000000004, "Y"=-29302.42}, {"X"=-0.03712, "Y"=-29302.42}, {"X"=-0.03404, "Y"=-29302.42}, {"X"=-0.03268, "Y"=-29302.42}, {"X"=-0.03148, "Y"=-29302.42}, {"X"=-0.02964, "Y"=-29302.42}, {"X"=-0.02784, "Y"=-29302.42}, {"X"=-0.027280000000000002, "Y"=-29302.42}, {"X"=-0.02648, "Y"=-29302.42}, {"X"=-0.02364, "Y"=-29302.42}, {"X"=-0.02288, "Y"=-29302.42}, {"X"=-0.0198, "Y"=-29302.42}, {"X"=-0.01924, "Y"=-29302.42}, {"X"=-0.0174, "Y"=-29302.42}, {"X"=-0.016, "Y"=-29302.42}, {"X"=-0.01344, "Y"=-29302.42}, {"X"=-0.011799999999999998, "Y"=-29302.42}, {"X"=-0.011439999999999999, "Y"=-29302.42}, {"X"=-0.009919999999999998, "Y"=-29302.42}, {"X"=-0.008559999999999998, "Y"=-29302.42}, {"X"=-0.007120000000000001, "Y"=-29302.42}, {"X"=-0.04616, "Y"=-27209.4}, {"X"=-0.04548, "Y"=-27209.4}, {"X"=-0.0422, "Y"=-27209.4}, {"X"=-0.04088, "Y"=-27209.4}, {"X"=-0.03884, "Y"=-27209.4}, {"X"=-0.03796, "Y"=-27209.4}, {"X"=-0.0378, "Y"=-27209.4}, {"X"=-0.03384, "Y"=-27209.4}, {"X"=-0.032600000000000004, "Y"=-27209.4}, {"X"=-0.031880000000000006, "Y"=-27209.4}, {"X"=-0.03144, "Y"=-27209.4}, {"X"=-0.02956, "Y"=-27209.4}, {"X"=-0.0274, "Y"=-27209.4}, {"X"=-0.02644, "Y"=-27209.4}, {"X"=-0.02348, "Y"=-27209.4}, {"X"=-0.02292, "Y"=-27209.4}, {"X"=-0.01968, "Y"=-27209.4}, {"X"=-0.01912, "Y"=-27209.4}, {"X"=-0.017320000000000002, "Y"=-27209.4}, {"X"=-0.016120000000000002, "Y"=-27209.4}, {"X"=-0.013400000000000002, "Y"=-27209.4}, {"X"=-0.011799999999999998, "Y"=-27209.4}, {"X"=-0.01004, "Y"=-27209.4}, {"X"=-0.009640000000000003, "Y"=-27209.4}, {"X"=-0.007679999999999999, "Y"=-27209.4}, {"X"=-0.0073599999999999985, "Y"=-27209.4}, {"X"=-0.006519999999999998, "Y"=-27209.4}, {"X"=-0.005080000000000001, "Y"=-27209.4}, {"X"=-0.04612, "Y"=-25116.379999999997}, {"X"=-0.045360000000000004, "Y"=-25116.379999999997}, {"X"=-0.04272, "Y"=-25116.379999999997}, {"X"=-0.041960000000000004, "Y"=-25116.379999999997}, {"X"=-0.04068, "Y"=-25116.379999999997}, {"X"=-0.04024, "Y"=-25116.379999999997}, {"X"=-0.03808, "Y"=-25116.379999999997}, {"X"=-0.037360000000000004, "Y"=-25116.379999999997}, {"X"=-0.03364, "Y"=-25116.379999999997}, {"X"=-0.03276, "Y"=-25116.379999999997}, {"X"=-0.03148, "Y"=-25116.379999999997}, {"X"=-0.0296, "Y"=-25116.379999999997}, {"X"=-0.027280000000000002, "Y"=-25116.379999999997}, {"X"=-0.02648, "Y"=-25116.379999999997}, {"X"=-0.02332, "Y"=-25116.379999999997}, {"X"=-0.01964, "Y"=-25116.379999999997}, {"X"=-0.01904, "Y"=-25116.379999999997}, {"X"=-0.017279999999999997, "Y"=-25116.379999999997}, {"X"=-0.016239999999999997, "Y"=-25116.379999999997}, {"X"=-0.01328, "Y"=-25116.379999999997}, {"X"=-0.011720000000000001, "Y"=-25116.379999999997}, {"X"=-0.010119999999999997, "Y"=-25116.379999999997}, {"X"=-0.009160000000000001, "Y"=-25116.379999999997}, {"X"=-0.008, "Y"=-25116.379999999997}, {"X"=-0.00716, "Y"=-25116.379999999997}, {"X"=-0.006399999999999996, "Y"=-25116.379999999997}, {"X"=-0.004839999999999997, "Y"=-25116.379999999997}, {"X"=-0.046360000000000005, "Y"=-23023.36}, {"X"=-0.04576, "Y"=-23023.36}, {"X"=-0.042120000000000005, "Y"=-23023.36}, {"X"=-0.04048, "Y"=-23023.36}, {"X"=-0.0396, "Y"=-23023.36}, {"X"=-0.03884, "Y"=-23023.36}, {"X"=-0.03756, "Y"=-23023.36}, {"X"=-0.03372, "Y"=-23023.36}, {"X"=-0.03296, "Y"=-23023.36}, {"X"=-0.03236, "Y"=-23023.36}, {"X"=-0.03096, "Y"=-23023.36}, {"X"=-0.02964, "Y"=-23023.36}, {"X"=-0.027200000000000002, "Y"=-23023.36}, {"X"=-0.02656, "Y"=-23023.36}, {"X"=-0.02324, "Y"=-23023.36}, {"X"=-0.0196, "Y"=-23023.36}, {"X"=-0.01912, "Y"=-23023.36}, {"X"=-0.017320000000000002, "Y"=-23023.36}, {"X"=-0.016399999999999998, "Y"=-23023.36}, {"X"=-0.013359999999999997, "Y"=-23023.36}, {"X"=-0.01192, "Y"=-23023.36}, {"X"=-0.00988, "Y"=-23023.36}, {"X"=-0.00936, "Y"=-23023.36}, {"X"=-0.00816, "Y"=-23023.36}, {"X"=-0.007280000000000002, "Y"=-23023.36}, {"X"=-0.006440000000000001, "Y"=-23023.36}, {"X"=-0.04576, "Y"=-20930.339999999997}, {"X"=-0.04512, "Y"=-20930.339999999997}, {"X"=-0.04224, "Y"=-20930.339999999997}, {"X"=-0.04164, "Y"=-20930.339999999997}, {"X"=-0.04032, "Y"=-20930.339999999997}, {"X"=-0.03828, "Y"=-20930.339999999997}, {"X"=-0.03752, "Y"=-20930.339999999997}, {"X"=-0.03352, "Y"=-20930.339999999997}, {"X"=-0.03172, "Y"=-20930.339999999997}, {"X"=-0.027440000000000003, "Y"=-20930.339999999997}, {"X"=-0.02684, "Y"=-20930.339999999997}, {"X"=-0.023280000000000002, "Y"=-20930.339999999997}, {"X"=-0.01928, "Y"=-20930.339999999997}, {"X"=-0.0174, "Y"=-20930.339999999997}, {"X"=-0.016599999999999997, "Y"=-20930.339999999997}, {"X"=-0.015399999999999997, "Y"=-20930.339999999997}, {"X"=-0.01344, "Y"=-20930.339999999997}, {"X"=-0.01208, "Y"=-20930.339999999997}, {"X"=-0.010239999999999999, "Y"=-20930.339999999997}, {"X"=-0.00988, "Y"=-20930.339999999997}, {"X"=-0.00936, "Y"=-20930.339999999997}, {"X"=-0.007960000000000002, "Y"=-20930.339999999997}, {"X"=-0.005600000000000001, "Y"=-20930.339999999997}, {"X"=-0.04528, "Y"=-18837.320000000007}, {"X"=-0.04168, "Y"=-18837.320000000007}, {"X"=-0.040040000000000006, "Y"=-18837.320000000007}, {"X"=-0.03864, "Y"=-18837.320000000007}, {"X"=-0.0382, "Y"=-18837.320000000007}, {"X"=-0.03744, "Y"=-18837.320000000007}, {"X"=-0.037200000000000004, "Y"=-18837.320000000007}, {"X"=-0.033280000000000004, "Y"=-18837.320000000007}, {"X"=-0.03208, "Y"=-18837.320000000007}, {"X"=-0.031560000000000005, "Y"=-18837.320000000007}, {"X"=-0.02756, "Y"=-18837.320000000007}, {"X"=-0.027, "Y"=-18837.320000000007}, {"X"=-0.02672, "Y"=-18837.320000000007}, {"X"=-0.02376, "Y"=-18837.320000000007}, {"X"=-0.02316, "Y"=-18837.320000000007}, {"X"=-0.01924, "Y"=-18837.320000000007}, {"X"=-0.017320000000000002, "Y"=-18837.320000000007}, {"X"=-0.016599999999999997, "Y"=-18837.320000000007}, {"X"=-0.015199999999999998, "Y"=-18837.320000000007}, {"X"=-0.013319999999999999, "Y"=-18837.320000000007}, {"X"=-0.012479999999999998, "Y"=-18837.320000000007}, {"X"=-0.011999999999999997, "Y"=-18837.320000000007}, {"X"=-0.010239999999999999, "Y"=-18837.320000000007}, {"X"=-0.009759999999999998, "Y"=-18837.320000000007}, {"X"=-0.00904, "Y"=-18837.320000000007}, {"X"=-0.00816, "Y"=-18837.320000000007}, {"X"=-0.005920000000000002, "Y"=-18837.320000000007}, {"X"=-0.045000000000000005, "Y"=-16744.300000000003}, {"X"=-0.041400000000000006, "Y"=-16744.300000000003}, {"X"=-0.03996, "Y"=-16744.300000000003}, {"X"=-0.03864, "Y"=-16744.300000000003}, {"X"=-0.038000000000000006, "Y"=-16744.300000000003}, {"X"=-0.03728, "Y"=-16744.300000000003}, {"X"=-0.03696, "Y"=-16744.300000000003}, {"X"=-0.03308, "Y"=-16744.300000000003}, {"X"=-0.032, "Y"=-16744.300000000003}, {"X"=-0.0314, "Y"=-16744.300000000003}, {"X"=-0.02692, "Y"=-16744.300000000003}, {"X"=-0.02636, "Y"=-16744.300000000003}, {"X"=-0.02364, "Y"=-16744.300000000003}, {"X"=-0.02304, "Y"=-16744.300000000003}, {"X"=-0.019200000000000002, "Y"=-16744.300000000003}, {"X"=-0.017279999999999997, "Y"=-16744.300000000003}, {"X"=-0.016640000000000002, "Y"=-16744.300000000003}, {"X"=-0.015199999999999998, "Y"=-16744.300000000003}, {"X"=-0.013240000000000002, "Y"=-16744.300000000003}, {"X"=-0.0126, "Y"=-16744.300000000003}, {"X"=-0.01208, "Y"=-16744.300000000003}, {"X"=-0.009959999999999997, "Y"=-16744.300000000003}, {"X"=-0.008919999999999997, "Y"=-16744.300000000003}, {"X"=-0.008399999999999998, "Y"=-16744.300000000003}, {"X"=-0.00648, "Y"=-16744.300000000003}, {"X"=-0.005240000000000002, "Y"=-16744.300000000003}, {"X"=-0.004799999999999999, "Y"=-16744.300000000003}, {"X"=-0.04532, "Y"=-14651.279999999999}, {"X"=-0.04476, "Y"=-14651.279999999999}, {"X"=-0.041800000000000004, "Y"=-14651.279999999999}, {"X"=-0.04124, "Y"=-14651.279999999999}, {"X"=-0.03964, "Y"=-14651.279999999999}, {"X"=-0.03832, "Y"=-14651.279999999999}, {"X"=-0.03724, "Y"=-14651.279999999999}, {"X"=-0.03312, "Y"=-14651.279999999999}, {"X"=-0.031560000000000005, "Y"=-14651.279999999999}, {"X"=-0.02752, "Y"=-14651.279999999999}, {"X"=-0.0268, "Y"=-14651.279999999999}, {"X"=-0.023200000000000002, "Y"=-14651.279999999999}, {"X"=-0.0194, "Y"=-14651.279999999999}, {"X"=-0.017439999999999997, "Y"=-14651.279999999999}, {"X"=-0.015440000000000002, "Y"=-14651.279999999999}, {"X"=-0.013479999999999999, "Y"=-14651.279999999999}, {"X"=-0.0126, "Y"=-14651.279999999999}, {"X"=-0.0104, "Y"=-14651.279999999999}, {"X"=-0.009559999999999999, "Y"=-14651.279999999999}, {"X"=-0.009239999999999998, "Y"=-14651.279999999999}, {"X"=-0.008480000000000001, "Y"=-14651.279999999999}, {"X"=-0.006159999999999999, "Y"=-14651.279999999999}, {"X"=-0.005400000000000002, "Y"=-14651.279999999999}, {"X"=-0.044840000000000005, "Y"=-12558.259999999995}, {"X"=-0.041760000000000005, "Y"=-12558.259999999995}, {"X"=-0.0412, "Y"=-12558.259999999995}, {"X"=-0.039720000000000005, "Y"=-12558.259999999995}, {"X"=-0.0388, "Y"=-12558.259999999995}, {"X"=-0.038000000000000006, "Y"=-12558.259999999995}, {"X"=-0.03724, "Y"=-12558.259999999995}, {"X"=-0.03672, "Y"=-12558.259999999995}, {"X"=-0.03276, "Y"=-12558.259999999995}, {"X"=-0.03136, "Y"=-12558.259999999995}, {"X"=-0.02808, "Y"=-12558.259999999995}, {"X"=-0.02696, "Y"=-12558.259999999995}, {"X"=-0.02648, "Y"=-12558.259999999995}, {"X"=-0.02344, "Y"=-12558.259999999995}, {"X"=-0.02304, "Y"=-12558.259999999995}, {"X"=-0.01932, "Y"=-12558.259999999995}, {"X"=-0.017320000000000002, "Y"=-12558.259999999995}, {"X"=-0.015359999999999999, "Y"=-12558.259999999995}, {"X"=-0.01328, "Y"=-12558.259999999995}, {"X"=-0.0126, "Y"=-12558.259999999995}, {"X"=-0.0104, "Y"=-12558.259999999995}, {"X"=-0.009279999999999997, "Y"=-12558.259999999995}, {"X"=-0.008599999999999997, "Y"=-12558.259999999995}, {"X"=-0.007960000000000002, "Y"=-12558.259999999995}, {"X"=-0.006199999999999997, "Y"=-12558.259999999995}, {"X"=-0.00476, "Y"=-12558.259999999995}, {"X"=-0.04464, "Y"=-10465.240000000005}, {"X"=-0.04308, "Y"=-10465.240000000005}, {"X"=-0.04132, "Y"=-10465.240000000005}, {"X"=-0.03948, "Y"=-10465.240000000005}, {"X"=-0.03844, "Y"=-10465.240000000005}, {"X"=-0.03696, "Y"=-10465.240000000005}, {"X"=-0.03248, "Y"=-10465.240000000005}, {"X"=-0.030080000000000003, "Y"=-10465.240000000005}, {"X"=-0.02764, "Y"=-10465.240000000005}, {"X"=-0.027280000000000002, "Y"=-10465.240000000005}, {"X"=-0.02656, "Y"=-10465.240000000005}, {"X"=-0.02352, "Y"=-10465.240000000005}, {"X"=-0.02304, "Y"=-10465.240000000005}, {"X"=-0.0194, "Y"=-10465.240000000005}, {"X"=-0.017640000000000003, "Y"=-10465.240000000005}, {"X"=-0.017120000000000003, "Y"=-10465.240000000005}, {"X"=-0.015440000000000002, "Y"=-10465.240000000005}, {"X"=-0.01312, "Y"=-10465.240000000005}, {"X"=-0.01228, "Y"=-10465.240000000005}, {"X"=-0.010360000000000001, "Y"=-10465.240000000005}, {"X"=-0.008919999999999997, "Y"=-10465.240000000005}, {"X"=-0.005839999999999998, "Y"=-10465.240000000005}, {"X"=-0.005319999999999998, "Y"=-10465.240000000005}, {"X"=-0.004880000000000002, "Y"=-10465.240000000005}, {"X"=-0.044520000000000004, "Y"=-8372.220000000001}, {"X"=-0.0432, "Y"=-8372.220000000001}, {"X"=-0.041120000000000004, "Y"=-8372.220000000001}, {"X"=-0.03932, "Y"=-8372.220000000001}, {"X"=-0.03812, "Y"=-8372.220000000001}, {"X"=-0.03676, "Y"=-8372.220000000001}, {"X"=-0.03268, "Y"=-8372.220000000001}, {"X"=-0.03228, "Y"=-8372.220000000001}, {"X"=-0.0314, "Y"=-8372.220000000001}, {"X"=-0.02996, "Y"=-8372.220000000001}, {"X"=-0.0268, "Y"=-8372.220000000001}, {"X"=-0.02316, "Y"=-8372.220000000001}, {"X"=-0.01932, "Y"=-8372.220000000001}, {"X"=-0.017279999999999997, "Y"=-8372.220000000001}, {"X"=-0.015280000000000002, "Y"=-8372.220000000001}, {"X"=-0.012999999999999998, "Y"=-8372.220000000001}, {"X"=-0.010160000000000002, "Y"=-8372.220000000001}, {"X"=-0.008960000000000003, "Y"=-8372.220000000001}, {"X"=-0.007600000000000003, "Y"=-8372.220000000001}, {"X"=-0.0056799999999999976, "Y"=-8372.220000000001}, {"X"=-0.005159999999999998, "Y"=-8372.220000000001}, {"X"=-0.0046, "Y"=-8372.220000000001}, {"X"=-0.04464, "Y"=-6279.199999999997}, {"X"=-0.043320000000000004, "Y"=-6279.199999999997}, {"X"=-0.0412, "Y"=-6279.199999999997}, {"X"=-0.03948, "Y"=-6279.199999999997}, {"X"=-0.03812, "Y"=-6279.199999999997}, {"X"=-0.03688, "Y"=-6279.199999999997}, {"X"=-0.032880000000000006, "Y"=-6279.199999999997}, {"X"=-0.031560000000000005, "Y"=-6279.199999999997}, {"X"=-0.030080000000000003, "Y"=-6279.199999999997}, {"X"=-0.02684, "Y"=-6279.199999999997}, {"X"=-0.023280000000000002, "Y"=-6279.199999999997}, {"X"=-0.01944, "Y"=-6279.199999999997}, {"X"=-0.017480000000000002, "Y"=-6279.199999999997}, {"X"=-0.015600000000000003, "Y"=-6279.199999999997}, {"X"=-0.01328, "Y"=-6279.199999999997}, {"X"=-0.01244, "Y"=-6279.199999999997}, {"X"=-0.010439999999999998, "Y"=-6279.199999999997}, {"X"=-0.009119999999999996, "Y"=-6279.199999999997}, {"X"=-0.005719999999999996, "Y"=-6279.199999999997}, {"X"=-0.005199999999999996, "Y"=-6279.199999999997}, {"X"=-0.04512, "Y"=-4186.180000000008}, {"X"=-0.0446, "Y"=-4186.180000000008}, {"X"=-0.04328, "Y"=-4186.180000000008}, {"X"=-0.04116, "Y"=-4186.180000000008}, {"X"=-0.03944, "Y"=-4186.180000000008}, {"X"=-0.03848, "Y"=-4186.180000000008}, {"X"=-0.037000000000000005, "Y"=-4186.180000000008}, {"X"=-0.032880000000000006, "Y"=-4186.180000000008}, {"X"=-0.03252, "Y"=-4186.180000000008}, {"X"=-0.03144, "Y"=-4186.180000000008}, {"X"=-0.030080000000000003, "Y"=-4186.180000000008}, {"X"=-0.027280000000000002, "Y"=-4186.180000000008}, {"X"=-0.026760000000000003, "Y"=-4186.180000000008}, {"X"=-0.02324, "Y"=-4186.180000000008}, {"X"=-0.01952, "Y"=-4186.180000000008}, {"X"=-0.017439999999999997, "Y"=-4186.180000000008}, {"X"=-0.015600000000000003, "Y"=-4186.180000000008}, {"X"=-0.013159999999999998, "Y"=-4186.180000000008}, {"X"=-0.012319999999999998, "Y"=-4186.180000000008}, {"X"=-0.010360000000000001, "Y"=-4186.180000000008}, {"X"=-0.009160000000000001, "Y"=-4186.180000000008}, {"X"=-0.005359999999999997, "Y"=-4186.180000000008}, {"X"=-0.04508, "Y"=-2093.1600000000035}, {"X"=-0.04344, "Y"=-2093.1600000000035}, {"X"=-0.041280000000000004, "Y"=-2093.1600000000035}, {"X"=-0.03952, "Y"=-2093.1600000000035}, {"X"=-0.03844, "Y"=-2093.1600000000035}, {"X"=-0.037040000000000003, "Y"=-2093.1600000000035}, {"X"=-0.032880000000000006, "Y"=-2093.1600000000035}, {"X"=-0.031520000000000006, "Y"=-2093.1600000000035}, {"X"=-0.030160000000000003, "Y"=-2093.1600000000035}, {"X"=-0.02708, "Y"=-2093.1600000000035}, {"X"=-0.02324, "Y"=-2093.1600000000035}, {"X"=-0.01952, "Y"=-2093.1600000000035}, {"X"=-0.017480000000000002, "Y"=-2093.1600000000035}, {"X"=-0.01564, "Y"=-2093.1600000000035}, {"X"=-0.013199999999999996, "Y"=-2093.1600000000035}, {"X"=-0.012360000000000003, "Y"=-2093.1600000000035}, {"X"=-0.010360000000000001, "Y"=-2093.1600000000035}, {"X"=-0.009160000000000001, "Y"=-2093.1600000000035}, {"X"=-0.005400000000000002, "Y"=-2093.1600000000035}, {"X"=-0.04488, "Y"=-0.13999999999941792}, {"X"=-0.0412, "Y"=-0.13999999999941792}, {"X"=-0.03956, "Y"=-0.13999999999941792}, {"X"=-0.038400000000000004, "Y"=-0.13999999999941792}, {"X"=-0.037040000000000003, "Y"=-0.13999999999941792}, {"X"=-0.032880000000000006, "Y"=-0.13999999999941792}, {"X"=-0.0316, "Y"=-0.13999999999941792}, {"X"=-0.030160000000000003, "Y"=-0.13999999999941792}, {"X"=-0.02696, "Y"=-0.13999999999941792}, {"X"=-0.02344, "Y"=-0.13999999999941792}, {"X"=-0.01952, "Y"=-0.13999999999941792}, {"X"=-0.017599999999999998, "Y"=-0.13999999999941792}, {"X"=-0.015760000000000003, "Y"=-0.13999999999941792}, {"X"=-0.013199999999999996, "Y"=-0.13999999999941792}, {"X"=-0.01244, "Y"=-0.13999999999941792}, {"X"=-0.010439999999999998, "Y"=-0.13999999999941792}, {"X"=-0.009160000000000001, "Y"=-0.13999999999941792}, {"X"=-0.005400000000000002, "Y"=-0.13999999999941792}, {"X"=-0.044680000000000004, "Y"=2092.8800000000047}, {"X"=-0.04116, "Y"=2092.8800000000047}, {"X"=-0.03952, "Y"=2092.8800000000047}, {"X"=-0.03808, "Y"=2092.8800000000047}, {"X"=-0.03684, "Y"=2092.8800000000047}, {"X"=-0.03296, "Y"=2092.8800000000047}, {"X"=-0.0316, "Y"=2092.8800000000047}, {"X"=-0.027, "Y"=2092.8800000000047}, {"X"=-0.0234, "Y"=2092.8800000000047}, {"X"=-0.01968, "Y"=2092.8800000000047}, {"X"=-0.017599999999999998, "Y"=2092.8800000000047}, {"X"=-0.015760000000000003, "Y"=2092.8800000000047}, {"X"=-0.013359999999999997, "Y"=2092.8800000000047}, {"X"=-0.012519999999999996, "Y"=2092.8800000000047}, {"X"=-0.01056, "Y"=2092.8800000000047}, {"X"=-0.00936, "Y"=2092.8800000000047}, {"X"=-0.00596, "Y"=2092.8800000000047}, {"X"=-0.005519999999999997, "Y"=2092.8800000000047}, {"X"=-0.044680000000000004, "Y"=4185.899999999994}, {"X"=-0.0434, "Y"=4185.899999999994}, {"X"=-0.04136, "Y"=4185.899999999994}, {"X"=-0.03956, "Y"=4185.899999999994}, {"X"=-0.038560000000000004, "Y"=4185.899999999994}, {"X"=-0.037040000000000003, "Y"=4185.899999999994}, {"X"=-0.03296, "Y"=4185.899999999994}, {"X"=-0.03264, "Y"=4185.899999999994}, {"X"=-0.031520000000000006, "Y"=4185.899999999994}, {"X"=-0.03088, "Y"=4185.899999999994}, {"X"=-0.02696, "Y"=4185.899999999994}, {"X"=-0.02344, "Y"=4185.899999999994}, {"X"=-0.01976, "Y"=4185.899999999994}, {"X"=-0.017640000000000003, "Y"=4185.899999999994}, {"X"=-0.015760000000000003, "Y"=4185.899999999994}, {"X"=-0.01344, "Y"=4185.899999999994}, {"X"=-0.012639999999999998, "Y"=4185.899999999994}, {"X"=-0.010639999999999997, "Y"=4185.899999999994}, {"X"=-0.009399999999999999, "Y"=4185.899999999994}, {"X"=-0.0061200000000000004, "Y"=4185.899999999994}, {"X"=-0.005600000000000001, "Y"=4185.899999999994}, {"X"=-0.04472, "Y"=6278.919999999998}, {"X"=-0.04116, "Y"=6278.919999999998}, {"X"=-0.03952, "Y"=6278.919999999998}, {"X"=-0.03812, "Y"=6278.919999999998}, {"X"=-0.03688, "Y"=6278.919999999998}, {"X"=-0.03296, "Y"=6278.919999999998}, {"X"=-0.0316, "Y"=6278.919999999998}, {"X"=-0.02696, "Y"=6278.919999999998}, {"X"=-0.0234, "Y"=6278.919999999998}, {"X"=-0.01972, "Y"=6278.919999999998}, {"X"=-0.017599999999999998, "Y"=6278.919999999998}, {"X"=-0.015760000000000003, "Y"=6278.919999999998}, {"X"=-0.013479999999999999, "Y"=6278.919999999998}, {"X"=-0.012720000000000002, "Y"=6278.919999999998}, {"X"=-0.010680000000000002, "Y"=6278.919999999998}, {"X"=-0.009480000000000002, "Y"=6278.919999999998}, {"X"=-0.006280000000000001, "Y"=6278.919999999998}, {"X"=-0.005760000000000001, "Y"=6278.919999999998}, {"X"=-0.004959999999999999, "Y"=6278.919999999998}, {"X"=-0.04936, "Y"=8371.940000000002}, {"X"=-0.044320000000000005, "Y"=8371.940000000002}, {"X"=-0.043000000000000003, "Y"=8371.940000000002}, {"X"=-0.041080000000000005, "Y"=8371.940000000002}, {"X"=-0.039240000000000004, "Y"=8371.940000000002}, {"X"=-0.03824, "Y"=8371.940000000002}, {"X"=-0.03676, "Y"=8371.940000000002}, {"X"=-0.03268, "Y"=8371.940000000002}, {"X"=-0.03228, "Y"=8371.940000000002}, {"X"=-0.030000000000000002, "Y"=8371.940000000002}, {"X"=-0.02708, "Y"=8371.940000000002}, {"X"=-0.026080000000000002, "Y"=8371.940000000002}, {"X"=-0.02312, "Y"=8371.940000000002}, {"X"=-0.01944, "Y"=8371.940000000002}, {"X"=-0.01736, "Y"=8371.940000000002}, {"X"=-0.01548, "Y"=8371.940000000002}, {"X"=-0.01328, "Y"=8371.940000000002}, {"X"=-0.012720000000000002, "Y"=8371.940000000002}, {"X"=-0.010439999999999998, "Y"=8371.940000000002}, {"X"=-0.0092, "Y"=8371.940000000002}, {"X"=-0.008320000000000001, "Y"=8371.940000000002}, {"X"=-0.005839999999999998, "Y"=8371.940000000002}, {"X"=-0.004959999999999999, "Y"=8371.940000000002}, {"X"=-0.04472, "Y"=10464.959999999992}, {"X"=-0.04328, "Y"=10464.959999999992}, {"X"=-0.04124, "Y"=10464.959999999992}, {"X"=-0.03952, "Y"=10464.959999999992}, {"X"=-0.03816, "Y"=10464.959999999992}, {"X"=-0.03688, "Y"=10464.959999999992}, {"X"=-0.033, "Y"=10464.959999999992}, {"X"=-0.03164, "Y"=10464.959999999992}, {"X"=-0.02704, "Y"=10464.959999999992}, {"X"=-0.02352, "Y"=10464.959999999992}, {"X"=-0.0198, "Y"=10464.959999999992}, {"X"=-0.01772, "Y"=10464.959999999992}, {"X"=-0.01588, "Y"=10464.959999999992}, {"X"=-0.013720000000000003, "Y"=10464.959999999992}, {"X"=-0.01296, "Y"=10464.959999999992}, {"X"=-0.01092, "Y"=10464.959999999992}, {"X"=-0.010119999999999997, "Y"=10464.959999999992}, {"X"=-0.009439999999999997, "Y"=10464.959999999992}, {"X"=-0.006519999999999998, "Y"=10464.959999999992}, {"X"=-0.005519999999999997, "Y"=10464.959999999992}, {"X"=-0.005039999999999996, "Y"=10464.959999999992}, {"X"=-0.04472, "Y"=12557.979999999996}, {"X"=-0.043320000000000004, "Y"=12557.979999999996}, {"X"=-0.041280000000000004, "Y"=12557.979999999996}, {"X"=-0.0396, "Y"=12557.979999999996}, {"X"=-0.03816, "Y"=12557.979999999996}, {"X"=-0.03692, "Y"=12557.979999999996}, {"X"=-0.03308, "Y"=12557.979999999996}, {"X"=-0.03164, "Y"=12557.979999999996}, {"X"=-0.02724, "Y"=12557.979999999996}, {"X"=-0.02684, "Y"=12557.979999999996}, {"X"=-0.02356, "Y"=12557.979999999996}, {"X"=-0.01984, "Y"=12557.979999999996}, {"X"=-0.01772, "Y"=12557.979999999996}, {"X"=-0.015919999999999997, "Y"=12557.979999999996}, {"X"=-0.013920000000000002, "Y"=12557.979999999996}, {"X"=-0.01296, "Y"=12557.979999999996}, {"X"=-0.011000000000000003, "Y"=12557.979999999996}, {"X"=-0.010239999999999999, "Y"=12557.979999999996}, {"X"=-0.00952, "Y"=12557.979999999996}, {"X"=-0.005319999999999998, "Y"=12557.979999999996}, {"X"=-0.04472, "Y"=14651.0}, {"X"=-0.04124, "Y"=14651.0}, {"X"=-0.03964, "Y"=14651.0}, {"X"=-0.03816, "Y"=14651.0}, {"X"=-0.03692, "Y"=14651.0}, {"X"=-0.03312, "Y"=14651.0}, {"X"=-0.03164, "Y"=14651.0}, {"X"=-0.028560000000000002, "Y"=14651.0}, {"X"=-0.02704, "Y"=14651.0}, {"X"=-0.0236, "Y"=14651.0}, {"X"=-0.0198, "Y"=14651.0}, {"X"=-0.01784, "Y"=14651.0}, {"X"=-0.015960000000000002, "Y"=14651.0}, {"X"=-0.014039999999999997, "Y"=14651.0}, {"X"=-0.012999999999999998, "Y"=14651.0}, {"X"=-0.011000000000000003, "Y"=14651.0}, {"X"=-0.01056, "Y"=14651.0}, {"X"=-0.009320000000000002, "Y"=14651.0}, {"X"=-0.00664, "Y"=14651.0}, {"X"=-0.00528, "Y"=14651.0}, {"X"=-0.0444, "Y"=16744.020000000004}, {"X"=-0.04104, "Y"=16744.020000000004}, {"X"=-0.03944, "Y"=16744.020000000004}, {"X"=-0.03808, "Y"=16744.020000000004}, {"X"=-0.03684, "Y"=16744.020000000004}, {"X"=-0.03312, "Y"=16744.020000000004}, {"X"=-0.031520000000000006, "Y"=16744.020000000004}, {"X"=-0.027200000000000002, "Y"=16744.020000000004}, {"X"=-0.02352, "Y"=16744.020000000004}, {"X"=-0.01964, "Y"=16744.020000000004}, {"X"=-0.01788, "Y"=16744.020000000004}, {"X"=-0.017279999999999997, "Y"=16744.020000000004}, {"X"=-0.01588, "Y"=16744.020000000004}, {"X"=-0.013999999999999999, "Y"=16744.020000000004}, {"X"=-0.012880000000000003, "Y"=16744.020000000004}, {"X"=-0.010639999999999997, "Y"=16744.020000000004}, {"X"=-0.009119999999999996, "Y"=16744.020000000004}, {"X"=-0.006559999999999996, "Y"=16744.020000000004}, {"X"=-0.00528, "Y"=16744.020000000004}, {"X"=-0.004839999999999997, "Y"=16744.020000000004}, {"X"=-0.044480000000000006, "Y"=18837.039999999994}, {"X"=-0.041120000000000004, "Y"=18837.039999999994}, {"X"=-0.039400000000000004, "Y"=18837.039999999994}, {"X"=-0.03816, "Y"=18837.039999999994}, {"X"=-0.03696, "Y"=18837.039999999994}, {"X"=-0.033240000000000006, "Y"=18837.039999999994}, {"X"=-0.031560000000000005, "Y"=18837.039999999994}, {"X"=-0.02972, "Y"=18837.039999999994}, {"X"=-0.027120000000000002, "Y"=18837.039999999994}, {"X"=-0.02356, "Y"=18837.039999999994}, {"X"=-0.01968, "Y"=18837.039999999994}, {"X"=-0.01792, "Y"=18837.039999999994}, {"X"=-0.0172, "Y"=18837.039999999994}, {"X"=-0.015919999999999997, "Y"=18837.039999999994}, {"X"=-0.014039999999999997, "Y"=18837.039999999994}, {"X"=-0.01276, "Y"=18837.039999999994}, {"X"=-0.010799999999999997, "Y"=18837.039999999994}, {"X"=-0.009959999999999997, "Y"=18837.039999999994}, {"X"=-0.008759999999999997, "Y"=18837.039999999994}, {"X"=-0.006999999999999999, "Y"=18837.039999999994}, {"X"=-0.006559999999999996, "Y"=18837.039999999994}, {"X"=-0.004799999999999999, "Y"=18837.039999999994}, {"X"=-0.044360000000000004, "Y"=20930.059999999998}, {"X"=-0.041120000000000004, "Y"=20930.059999999998}, {"X"=-0.0396, "Y"=20930.059999999998}, {"X"=-0.03816, "Y"=20930.059999999998}, {"X"=-0.03696, "Y"=20930.059999999998}, {"X"=-0.033280000000000004, "Y"=20930.059999999998}, {"X"=-0.031520000000000006, "Y"=20930.059999999998}, {"X"=-0.02964, "Y"=20930.059999999998}, {"X"=-0.02692, "Y"=20930.059999999998}, {"X"=-0.02352, "Y"=20930.059999999998}, {"X"=-0.0196, "Y"=20930.059999999998}, {"X"=-0.01792, "Y"=20930.059999999998}, {"X"=-0.017079999999999998, "Y"=20930.059999999998}, {"X"=-0.0158, "Y"=20930.059999999998}, {"X"=-0.014039999999999997, "Y"=20930.059999999998}, {"X"=-0.012639999999999998, "Y"=20930.059999999998}, {"X"=-0.01092, "Y"=20930.059999999998}, {"X"=-0.010479999999999996, "Y"=20930.059999999998}, {"X"=-0.008800000000000002, "Y"=20930.059999999998}, {"X"=-0.00784, "Y"=20930.059999999998}, {"X"=-0.0448, "Y"=23023.08}, {"X"=-0.041280000000000004, "Y"=23023.08}, {"X"=-0.039760000000000004, "Y"=23023.08}, {"X"=-0.03844, "Y"=23023.08}, {"X"=-0.037000000000000005, "Y"=23023.08}, {"X"=-0.0334, "Y"=23023.08}, {"X"=-0.03248, "Y"=23023.08}, {"X"=-0.031520000000000006, "Y"=23023.08}, {"X"=-0.0296, "Y"=23023.08}, {"X"=-0.027120000000000002, "Y"=23023.08}, {"X"=-0.0236, "Y"=23023.08}, {"X"=-0.0196, "Y"=23023.08}, {"X"=-0.017959999999999997, "Y"=23023.08}, {"X"=-0.01688, "Y"=23023.08}, {"X"=-0.01412, "Y"=23023.08}, {"X"=-0.0126, "Y"=23023.08}, {"X"=-0.010639999999999997, "Y"=23023.08}, {"X"=-0.009000000000000001, "Y"=23023.08}, {"X"=-0.008039999999999999, "Y"=23023.08}, {"X"=-0.007600000000000003, "Y"=23023.08}, {"X"=-0.006039999999999997, "Y"=23023.08}, {"X"=-0.004679999999999997, "Y"=23023.08}, {"X"=-0.04492, "Y"=25116.100000000006}, {"X"=-0.04136, "Y"=25116.100000000006}, {"X"=-0.0398, "Y"=25116.100000000006}, {"X"=-0.03916, "Y"=25116.100000000006}, {"X"=-0.038680000000000006, "Y"=25116.100000000006}, {"X"=-0.03708, "Y"=25116.100000000006}, {"X"=-0.03352, "Y"=25116.100000000006}, {"X"=-0.03272, "Y"=25116.100000000006}, {"X"=-0.03196, "Y"=25116.100000000006}, {"X"=-0.02956, "Y"=25116.100000000006}, {"X"=-0.027280000000000002, "Y"=25116.100000000006}, {"X"=-0.02644, "Y"=25116.100000000006}, {"X"=-0.0236, "Y"=25116.100000000006}, {"X"=-0.019960000000000002, "Y"=25116.100000000006}, {"X"=-0.01948, "Y"=25116.100000000006}, {"X"=-0.01788, "Y"=25116.100000000006}, {"X"=-0.01656, "Y"=25116.100000000006}, {"X"=-0.014039999999999997, "Y"=25116.100000000006}, {"X"=-0.01244, "Y"=25116.100000000006}, {"X"=-0.010799999999999997, "Y"=25116.100000000006}, {"X"=-0.010520000000000002, "Y"=25116.100000000006}, {"X"=-0.008, "Y"=25116.100000000006}, {"X"=-0.006159999999999999, "Y"=25116.100000000006}, {"X"=-0.04508, "Y"=27209.119999999995}, {"X"=-0.04156, "Y"=27209.119999999995}, {"X"=-0.04012, "Y"=27209.119999999995}, {"X"=-0.03912, "Y"=27209.119999999995}, {"X"=-0.037200000000000004, "Y"=27209.119999999995}, {"X"=-0.0358, "Y"=27209.119999999995}, {"X"=-0.0338, "Y"=27209.119999999995}, {"X"=-0.03316, "Y"=27209.119999999995}, {"X"=-0.03228, "Y"=27209.119999999995}, {"X"=-0.031, "Y"=27209.119999999995}, {"X"=-0.0298, "Y"=27209.119999999995}, {"X"=-0.02732, "Y"=27209.119999999995}, {"X"=-0.026680000000000002, "Y"=27209.119999999995}, {"X"=-0.02624, "Y"=27209.119999999995}, {"X"=-0.02372, "Y"=27209.119999999995}, {"X"=-0.02028, "Y"=27209.119999999995}, {"X"=-0.0198, "Y"=27209.119999999995}, {"X"=-0.01928, "Y"=27209.119999999995}, {"X"=-0.01784, "Y"=27209.119999999995}, {"X"=-0.016759999999999997, "Y"=27209.119999999995}, {"X"=-0.01412, "Y"=27209.119999999995}, {"X"=-0.012319999999999998, "Y"=27209.119999999995}, {"X"=-0.010680000000000002, "Y"=27209.119999999995}, {"X"=-0.008320000000000001, "Y"=27209.119999999995}, {"X"=-0.0074800000000000005, "Y"=27209.119999999995}, {"X"=-0.0456, "Y"=29302.14}, {"X"=-0.04524, "Y"=29302.14}, {"X"=-0.044480000000000006, "Y"=29302.14}, {"X"=-0.04164, "Y"=29302.14}, {"X"=-0.04028, "Y"=29302.14}, {"X"=-0.03932, "Y"=29302.14}, {"X"=-0.03844, "Y"=29302.14}, {"X"=-0.037360000000000004, "Y"=29302.14}, {"X"=-0.03616, "Y"=29302.14}, {"X"=-0.03372, "Y"=29302.14}, {"X"=-0.03236, "Y"=29302.14}, {"X"=-0.03128, "Y"=29302.14}, {"X"=-0.029480000000000003, "Y"=29302.14}, {"X"=-0.02752, "Y"=29302.14}, {"X"=-0.026520000000000002, "Y"=29302.14}, {"X"=-0.023880000000000002, "Y"=29302.14}, {"X"=-0.02312, "Y"=29302.14}, {"X"=-0.02032, "Y"=29302.14}, {"X"=-0.01944, "Y"=29302.14}, {"X"=-0.019, "Y"=29302.14}, {"X"=-0.017959999999999997, "Y"=29302.14}, {"X"=-0.01652, "Y"=29302.14}, {"X"=-0.01412, "Y"=29302.14}, {"X"=-0.012400000000000001, "Y"=29302.14}, {"X"=-0.01208, "Y"=29302.14}, {"X"=-0.010959999999999998, "Y"=29302.14}, {"X"=-0.009799999999999996, "Y"=29302.14}, {"X"=-0.008079999999999997, "Y"=29302.14}, {"X"=-0.007800000000000001, "Y"=29302.14}, {"X"=-0.007399999999999997, "Y"=29302.14}, {"X"=-0.005760000000000001, "Y"=29302.14}, {"X"=-0.005240000000000002, "Y"=29302.14}, {"X"=-0.004839999999999997, "Y"=29302.14}, {"X"=-0.045680000000000005, "Y"=31395.160000000003}, {"X"=-0.044840000000000005, "Y"=31395.160000000003}, {"X"=-0.04192, "Y"=31395.160000000003}, {"X"=-0.041400000000000006, "Y"=31395.160000000003}, {"X"=-0.0402, "Y"=31395.160000000003}, {"X"=-0.038680000000000006, "Y"=31395.160000000003}, {"X"=-0.037720000000000004, "Y"=31395.160000000003}, {"X"=-0.037360000000000004, "Y"=31395.160000000003}, {"X"=-0.036640000000000006, "Y"=31395.160000000003}, {"X"=-0.03388, "Y"=31395.160000000003}, {"X"=-0.03244, "Y"=31395.160000000003}, {"X"=-0.03132, "Y"=31395.160000000003}, {"X"=-0.02956, "Y"=31395.160000000003}, {"X"=-0.02772, "Y"=31395.160000000003}, {"X"=-0.026600000000000002, "Y"=31395.160000000003}, {"X"=-0.02408, "Y"=31395.160000000003}, {"X"=-0.02316, "Y"=31395.160000000003}, {"X"=-0.02052, "Y"=31395.160000000003}, {"X"=-0.01984, "Y"=31395.160000000003}, {"X"=-0.01928, "Y"=31395.160000000003}, {"X"=-0.01808, "Y"=31395.160000000003}, {"X"=-0.01652, "Y"=31395.160000000003}, {"X"=-0.014240000000000003, "Y"=31395.160000000003}, {"X"=-0.012119999999999999, "Y"=31395.160000000003}, {"X"=-0.008039999999999999, "Y"=31395.160000000003}, {"X"=-0.005639999999999999, "Y"=31395.160000000003}, {"X"=-0.0049999999999999975, "Y"=31395.160000000003}, {"X"=-0.046040000000000005, "Y"=33488.17999999999}, {"X"=-0.04512, "Y"=33488.17999999999}, {"X"=-0.042, "Y"=33488.17999999999}, {"X"=-0.041440000000000005, "Y"=33488.17999999999}, {"X"=-0.04032, "Y"=33488.17999999999}, {"X"=-0.0398, "Y"=33488.17999999999}, {"X"=-0.03888, "Y"=33488.17999999999}, {"X"=-0.0374, "Y"=33488.17999999999}, {"X"=-0.03672, "Y"=33488.17999999999}, {"X"=-0.033920000000000006, "Y"=33488.17999999999}, {"X"=-0.03232, "Y"=33488.17999999999}, {"X"=-0.03108, "Y"=33488.17999999999}, {"X"=-0.029400000000000003, "Y"=33488.17999999999}, {"X"=-0.02772, "Y"=33488.17999999999}, {"X"=-0.02724, "Y"=33488.17999999999}, {"X"=-0.02636, "Y"=33488.17999999999}, {"X"=-0.024, "Y"=33488.17999999999}, {"X"=-0.02292, "Y"=33488.17999999999}, {"X"=-0.020560000000000002, "Y"=33488.17999999999}, {"X"=-0.01884, "Y"=33488.17999999999}, {"X"=-0.01788, "Y"=33488.17999999999}, {"X"=-0.0162, "Y"=33488.17999999999}, {"X"=-0.014159999999999999, "Y"=33488.17999999999}, {"X"=-0.011959999999999998, "Y"=33488.17999999999}, {"X"=-0.010799999999999997, "Y"=33488.17999999999}, {"X"=-0.008079999999999997, "Y"=33488.17999999999}, {"X"=-0.007800000000000001, "Y"=33488.17999999999}, {"X"=-0.00648, "Y"=33488.17999999999}, {"X"=-0.005240000000000002, "Y"=33488.17999999999}, {"X"=-0.004799999999999999, "Y"=33488.17999999999}, {"X"=-0.04592, "Y"=35581.2}, {"X"=-0.044840000000000005, "Y"=35581.2}, {"X"=-0.0422, "Y"=35581.2}, {"X"=-0.041400000000000006, "Y"=35581.2}, {"X"=-0.040080000000000005, "Y"=35581.2}, {"X"=-0.039240000000000004, "Y"=35581.2}, {"X"=-0.03892, "Y"=35581.2}, {"X"=-0.037880000000000004, "Y"=35581.2}, {"X"=-0.037320000000000006, "Y"=35581.2}, {"X"=-0.0366, "Y"=35581.2}, {"X"=-0.03408, "Y"=35581.2}, {"X"=-0.0324, "Y"=35581.2}, {"X"=-0.03124, "Y"=35581.2}, {"X"=-0.02944, "Y"=35581.2}, {"X"=-0.02768, "Y"=35581.2}, {"X"=-0.0264, "Y"=35581.2}, {"X"=-0.02424, "Y"=35581.2}, {"X"=-0.02296, "Y"=35581.2}, {"X"=-0.02076, "Y"=35581.2}, {"X"=-0.019880000000000002, "Y"=35581.2}, {"X"=-0.019, "Y"=35581.2}, {"X"=-0.01804, "Y"=35581.2}, {"X"=-0.0162, "Y"=35581.2}, {"X"=-0.014400000000000003, "Y"=35581.2}, {"X"=-0.01208, "Y"=35581.2}, {"X"=-0.01088, "Y"=35581.2}, {"X"=-0.00836, "Y"=35581.2}, {"X"=-0.007919999999999996, "Y"=35581.2}, {"X"=-0.006559999999999996, "Y"=35581.2}, {"X"=-0.006159999999999999, "Y"=35581.2}, {"X"=-0.005080000000000001, "Y"=35581.2}, {"X"=-0.004679999999999997, "Y"=35581.2}, {"X"=-0.046040000000000005, "Y"=37674.22}, {"X"=-0.044840000000000005, "Y"=37674.22}, {"X"=-0.042280000000000005, "Y"=37674.22}, {"X"=-0.04136, "Y"=37674.22}, {"X"=-0.040600000000000004, "Y"=37674.22}, {"X"=-0.03988, "Y"=37674.22}, {"X"=-0.039040000000000005, "Y"=37674.22}, {"X"=-0.037880000000000004, "Y"=37674.22}, {"X"=-0.03724, "Y"=37674.22}, {"X"=-0.03404, "Y"=37674.22}, {"X"=-0.032200000000000006, "Y"=37674.22}, {"X"=-0.03108, "Y"=37674.22}, {"X"=-0.0292, "Y"=37674.22}, {"X"=-0.02772, "Y"=37674.22}, {"X"=-0.026600000000000002, "Y"=37674.22}, {"X"=-0.026080000000000002, "Y"=37674.22}, {"X"=-0.02412, "Y"=37674.22}, {"X"=-0.02264, "Y"=37674.22}, {"X"=-0.020640000000000002, "Y"=37674.22}, {"X"=-0.01972, "Y"=37674.22}, {"X"=-0.018639999999999997, "Y"=37674.22}, {"X"=-0.01784, "Y"=37674.22}, {"X"=-0.015760000000000003, "Y"=37674.22}, {"X"=-0.014280000000000001, "Y"=37674.22}, {"X"=-0.012319999999999998, "Y"=37674.22}, {"X"=-0.011520000000000002, "Y"=37674.22}, {"X"=-0.0104, "Y"=37674.22}, {"X"=-0.008399999999999998, "Y"=37674.22}, {"X"=-0.007759999999999996, "Y"=37674.22}, {"X"=-0.0062400000000000025, "Y"=37674.22}, {"X"=-0.0056799999999999976, "Y"=37674.22}, {"X"=-0.04592, "Y"=39767.240000000005}, {"X"=-0.044520000000000004, "Y"=39767.240000000005}, {"X"=-0.04268, "Y"=39767.240000000005}, {"X"=-0.042, "Y"=39767.240000000005}, {"X"=-0.041080000000000005, "Y"=39767.240000000005}, {"X"=-0.04024, "Y"=39767.240000000005}, {"X"=-0.03944, "Y"=39767.240000000005}, {"X"=-0.039040000000000005, "Y"=39767.240000000005}, {"X"=-0.037880000000000004, "Y"=39767.240000000005}, {"X"=-0.03724, "Y"=39767.240000000005}, {"X"=-0.036680000000000004, "Y"=39767.240000000005}, {"X"=-0.03412, "Y"=39767.240000000005}, {"X"=-0.03248, "Y"=39767.240000000005}, {"X"=-0.03104, "Y"=39767.240000000005}, {"X"=-0.02912, "Y"=39767.240000000005}, {"X"=-0.02772, "Y"=39767.240000000005}, {"X"=-0.02596, "Y"=39767.240000000005}, {"X"=-0.0242, "Y"=39767.240000000005}, {"X"=-0.022520000000000002, "Y"=39767.240000000005}, {"X"=-0.02044, "Y"=39767.240000000005}, {"X"=-0.0186, "Y"=39767.240000000005}, {"X"=-0.01788, "Y"=39767.240000000005}, {"X"=-0.01564, "Y"=39767.240000000005}, {"X"=-0.014400000000000003, "Y"=39767.240000000005}, {"X"=-0.012639999999999998, "Y"=39767.240000000005}, {"X"=-0.012040000000000002, "Y"=39767.240000000005}, {"X"=-0.011319999999999997, "Y"=39767.240000000005}, {"X"=-0.011000000000000003, "Y"=39767.240000000005}, {"X"=-0.010520000000000002, "Y"=39767.240000000005}, {"X"=-0.00884, "Y"=39767.240000000005}, {"X"=-0.007800000000000001, "Y"=39767.240000000005}, {"X"=-0.00664, "Y"=39767.240000000005}, {"X"=-0.004519999999999996, "Y"=39767.240000000005}, {"X"=-0.0466, "Y"=41860.26000000001}, {"X"=-0.045200000000000004, "Y"=41860.26000000001}, {"X"=-0.04252, "Y"=41860.26000000001}, {"X"=-0.041440000000000005, "Y"=41860.26000000001}, {"X"=-0.03984, "Y"=41860.26000000001}, {"X"=-0.03932, "Y"=41860.26000000001}, {"X"=-0.03816, "Y"=41860.26000000001}, {"X"=-0.03692, "Y"=41860.26000000001}, {"X"=-0.034280000000000005, "Y"=41860.26000000001}, {"X"=-0.0334, "Y"=41860.26000000001}, {"X"=-0.03184, "Y"=41860.26000000001}, {"X"=-0.03108, "Y"=41860.26000000001}, {"X"=-0.02908, "Y"=41860.26000000001}, {"X"=-0.02776, "Y"=41860.26000000001}, {"X"=-0.0258, "Y"=41860.26000000001}, {"X"=-0.02424, "Y"=41860.26000000001}, {"X"=-0.0228, "Y"=41860.26000000001}, {"X"=-0.02224, "Y"=41860.26000000001}, {"X"=-0.02024, "Y"=41860.26000000001}, {"X"=-0.018279999999999998, "Y"=41860.26000000001}, {"X"=-0.015239999999999997, "Y"=41860.26000000001}, {"X"=-0.014359999999999998, "Y"=41860.26000000001}, {"X"=-0.012360000000000003, "Y"=41860.26000000001}, {"X"=-0.011200000000000002, "Y"=41860.26000000001}, {"X"=-0.010599999999999998, "Y"=41860.26000000001}, {"X"=-0.0102, "Y"=41860.26000000001}, {"X"=-0.008, "Y"=41860.26000000001}, {"X"=-0.007199999999999998, "Y"=41860.26000000001}, {"X"=-0.006280000000000001, "Y"=41860.26000000001}, {"X"=-0.004920000000000001, "Y"=41860.26000000001}, {"X"=-0.04664, "Y"=43953.28}, {"X"=-0.04512, "Y"=43953.28}, {"X"=-0.042640000000000004, "Y"=43953.28}, {"X"=-0.04104, "Y"=43953.28}, {"X"=-0.03996, "Y"=43953.28}, {"X"=-0.03944, "Y"=43953.28}, {"X"=-0.039040000000000005, "Y"=43953.28}, {"X"=-0.03828, "Y"=43953.28}, {"X"=-0.03692, "Y"=43953.28}, {"X"=-0.034280000000000005, "Y"=43953.28}, {"X"=-0.03344, "Y"=43953.28}, {"X"=-0.031920000000000004, "Y"=43953.28}, {"X"=-0.03132, "Y"=43953.28}, {"X"=-0.02908, "Y"=43953.28}, {"X"=-0.02784, "Y"=43953.28}, {"X"=-0.026080000000000002, "Y"=43953.28}, {"X"=-0.02556, "Y"=43953.28}, {"X"=-0.02424, "Y"=43953.28}, {"X"=-0.02232, "Y"=43953.28}, {"X"=-0.0202, "Y"=43953.28}, {"X"=-0.01836, "Y"=43953.28}, {"X"=-0.01784, "Y"=43953.28}, {"X"=-0.01516, "Y"=43953.28}, {"X"=-0.01432, "Y"=43953.28}, {"X"=-0.012319999999999998, "Y"=43953.28}, {"X"=-0.011279999999999998, "Y"=43953.28}, {"X"=-0.01072, "Y"=43953.28}, {"X"=-0.0104, "Y"=43953.28}, {"X"=-0.007399999999999997, "Y"=43953.28}, {"X"=-0.004679999999999997, "Y"=43953.28}, {"X"=-0.04676, "Y"=46046.29999999999}, {"X"=-0.04612, "Y"=46046.29999999999}, {"X"=-0.04524, "Y"=46046.29999999999}, {"X"=-0.0444, "Y"=46046.29999999999}, {"X"=-0.04268, "Y"=46046.29999999999}, {"X"=-0.04096, "Y"=46046.29999999999}, {"X"=-0.040080000000000005, "Y"=46046.29999999999}, {"X"=-0.0396, "Y"=46046.29999999999}, {"X"=-0.0392, "Y"=46046.29999999999}, {"X"=-0.0382, "Y"=46046.29999999999}, {"X"=-0.03776, "Y"=46046.29999999999}, {"X"=-0.037040000000000003, "Y"=46046.29999999999}, {"X"=-0.03432, "Y"=46046.29999999999}, {"X"=-0.03352, "Y"=46046.29999999999}, {"X"=-0.03184, "Y"=46046.29999999999}, {"X"=-0.028, "Y"=46046.29999999999}, {"X"=-0.02756, "Y"=46046.29999999999}, {"X"=-0.02636, "Y"=46046.29999999999}, {"X"=-0.02568, "Y"=46046.29999999999}, {"X"=-0.02424, "Y"=46046.29999999999}, {"X"=-0.02224, "Y"=46046.29999999999}, {"X"=-0.019960000000000002, "Y"=46046.29999999999}, {"X"=-0.01788, "Y"=46046.29999999999}, {"X"=-0.01448, "Y"=46046.29999999999}, {"X"=-0.012240000000000001, "Y"=46046.29999999999}, {"X"=-0.010360000000000001, "Y"=46046.29999999999}, {"X"=-0.007559999999999997, "Y"=46046.29999999999}, {"X"=-0.007120000000000001, "Y"=46046.29999999999}, {"X"=-0.0062400000000000025, "Y"=46046.29999999999}, {"X"=-0.046720000000000005, "Y"=48139.32000000001}, {"X"=-0.04496, "Y"=48139.32000000001}, {"X"=-0.04288, "Y"=48139.32000000001}, {"X"=-0.041440000000000005, "Y"=48139.32000000001}, {"X"=-0.03964, "Y"=48139.32000000001}, {"X"=-0.03864, "Y"=48139.32000000001}, {"X"=-0.038360000000000005, "Y"=48139.32000000001}, {"X"=-0.037680000000000005, "Y"=48139.32000000001}, {"X"=-0.0366, "Y"=48139.32000000001}, {"X"=-0.034480000000000004, "Y"=48139.32000000001}, {"X"=-0.0328, "Y"=48139.32000000001}, {"X"=-0.0314, "Y"=48139.32000000001}, {"X"=-0.028, "Y"=48139.32000000001}, {"X"=-0.02576, "Y"=48139.32000000001}, {"X"=-0.024480000000000002, "Y"=48139.32000000001}, {"X"=-0.02224, "Y"=48139.32000000001}, {"X"=-0.02016, "Y"=48139.32000000001}, {"X"=-0.01808, "Y"=48139.32000000001}, {"X"=-0.0148, "Y"=48139.32000000001}, {"X"=-0.01228, "Y"=48139.32000000001}, {"X"=-0.010799999999999997, "Y"=48139.32000000001}, {"X"=-0.008079999999999997, "Y"=48139.32000000001}, {"X"=-0.007519999999999999, "Y"=48139.32000000001}, {"X"=-0.0066799999999999984, "Y"=48139.32000000001}, {"X"=-0.006039999999999997, "Y"=48139.32000000001}, {"X"=-0.0056799999999999976, "Y"=48139.32000000001}, {"X"=-0.004880000000000002, "Y"=48139.32000000001}, {"X"=-0.04716, "Y"=50232.34}, {"X"=-0.04644, "Y"=50232.34}, {"X"=-0.045360000000000004, "Y"=50232.34}, {"X"=-0.043120000000000006, "Y"=50232.34}, {"X"=-0.04156, "Y"=50232.34}, {"X"=-0.040400000000000005, "Y"=50232.34}, {"X"=-0.03996, "Y"=50232.34}, {"X"=-0.038720000000000004, "Y"=50232.34}, {"X"=-0.03684, "Y"=50232.34}, {"X"=-0.03548, "Y"=50232.34}, {"X"=-0.03452, "Y"=50232.34}, {"X"=-0.03284, "Y"=50232.34}, {"X"=-0.03148, "Y"=50232.34}, {"X"=-0.028, "Y"=50232.34}, {"X"=-0.0256, "Y"=50232.34}, {"X"=-0.024480000000000002, "Y"=50232.34}, {"X"=-0.02204, "Y"=50232.34}, {"X"=-0.02, "Y"=50232.34}, {"X"=-0.01824, "Y"=50232.34}, {"X"=-0.016640000000000002, "Y"=50232.34}, {"X"=-0.014760000000000002, "Y"=50232.34}, {"X"=-0.012400000000000001, "Y"=50232.34}, {"X"=-0.010639999999999997, "Y"=50232.34}, {"X"=-0.007640000000000001, "Y"=50232.34}, {"X"=-0.0074800000000000005, "Y"=50232.34}, {"X"=-0.006960000000000001, "Y"=50232.34}, {"X"=-0.005600000000000001, "Y"=50232.34}, {"X"=-0.04664, "Y"=52325.359999999986}, {"X"=-0.04528, "Y"=52325.359999999986}, {"X"=-0.04308, "Y"=52325.359999999986}, {"X"=-0.041440000000000005, "Y"=52325.359999999986}, {"X"=-0.04036, "Y"=52325.359999999986}, {"X"=-0.03952, "Y"=52325.359999999986}, {"X"=-0.039080000000000004, "Y"=52325.359999999986}, {"X"=-0.0386, "Y"=52325.359999999986}, {"X"=-0.0376, "Y"=52325.359999999986}, {"X"=-0.036680000000000004, "Y"=52325.359999999986}, {"X"=-0.03572, "Y"=52325.359999999986}, {"X"=-0.03456, "Y"=52325.359999999986}, {"X"=-0.03304, "Y"=52325.359999999986}, {"X"=-0.03148, "Y"=52325.359999999986}, {"X"=-0.03036, "Y"=52325.359999999986}, {"X"=-0.028040000000000002, "Y"=52325.359999999986}, {"X"=-0.027200000000000002, "Y"=52325.359999999986}, {"X"=-0.02544, "Y"=52325.359999999986}, {"X"=-0.02452, "Y"=52325.359999999986}, {"X"=-0.02188, "Y"=52325.359999999986}, {"X"=-0.02004, "Y"=52325.359999999986}, {"X"=-0.018279999999999998, "Y"=52325.359999999986}, {"X"=-0.01652, "Y"=52325.359999999986}, {"X"=-0.01448, "Y"=52325.359999999986}, {"X"=-0.01244, "Y"=52325.359999999986}, {"X"=-0.01056, "Y"=52325.359999999986}, {"X"=-0.007519999999999999, "Y"=52325.359999999986}, {"X"=-0.005839999999999998, "Y"=52325.359999999986}, {"X"=-0.005519999999999997, "Y"=52325.359999999986}, {"X"=-0.04664, "Y"=54418.380000000005}, {"X"=-0.04456, "Y"=54418.380000000005}, {"X"=-0.04288, "Y"=54418.380000000005}, {"X"=-0.041080000000000005, "Y"=54418.380000000005}, {"X"=-0.040080000000000005, "Y"=54418.380000000005}, {"X"=-0.03964, "Y"=54418.380000000005}, {"X"=-0.038720000000000004, "Y"=54418.380000000005}, {"X"=-0.03748, "Y"=54418.380000000005}, {"X"=-0.03628, "Y"=54418.380000000005}, {"X"=-0.03456, "Y"=54418.380000000005}, {"X"=-0.032920000000000005, "Y"=54418.380000000005}, {"X"=-0.031520000000000006, "Y"=54418.380000000005}, {"X"=-0.03028, "Y"=54418.380000000005}, {"X"=-0.028120000000000003, "Y"=54418.380000000005}, {"X"=-0.027200000000000002, "Y"=54418.380000000005}, {"X"=-0.025400000000000002, "Y"=54418.380000000005}, {"X"=-0.0246, "Y"=54418.380000000005}, {"X"=-0.02176, "Y"=54418.380000000005}, {"X"=-0.02012, "Y"=54418.380000000005}, {"X"=-0.018279999999999998, "Y"=54418.380000000005}, {"X"=-0.016640000000000002, "Y"=54418.380000000005}, {"X"=-0.01448, "Y"=54418.380000000005}, {"X"=-0.0126, "Y"=54418.380000000005}, {"X"=-0.010479999999999996, "Y"=54418.380000000005}, {"X"=-0.008399999999999998, "Y"=54418.380000000005}, {"X"=-0.007879999999999998, "Y"=54418.380000000005}, {"X"=-0.007440000000000002, "Y"=54418.380000000005}, {"X"=-0.005920000000000002, "Y"=54418.380000000005}, {"X"=-0.005319999999999998, "Y"=54418.380000000005}, {"X"=-0.004880000000000002, "Y"=54418.380000000005}, {"X"=-0.04732, "Y"=56511.399999999994}, {"X"=-0.04528, "Y"=56511.399999999994}, {"X"=-0.0434, "Y"=56511.399999999994}, {"X"=-0.04148, "Y"=56511.399999999994}, {"X"=-0.04064, "Y"=56511.399999999994}, {"X"=-0.0398, "Y"=56511.399999999994}, {"X"=-0.03876, "Y"=56511.399999999994}, {"X"=-0.037680000000000005, "Y"=56511.399999999994}, {"X"=-0.037200000000000004, "Y"=56511.399999999994}, {"X"=-0.03644, "Y"=56511.399999999994}, {"X"=-0.03476, "Y"=56511.399999999994}, {"X"=-0.03304, "Y"=56511.399999999994}, {"X"=-0.03168, "Y"=56511.399999999994}, {"X"=-0.0304, "Y"=56511.399999999994}, {"X"=-0.02836, "Y"=56511.399999999994}, {"X"=-0.02768, "Y"=56511.399999999994}, {"X"=-0.02548, "Y"=56511.399999999994}, {"X"=-0.02484, "Y"=56511.399999999994}, {"X"=-0.021840000000000002, "Y"=56511.399999999994}, {"X"=-0.0204, "Y"=56511.399999999994}, {"X"=-0.018480000000000003, "Y"=56511.399999999994}, {"X"=-0.016759999999999997, "Y"=56511.399999999994}, {"X"=-0.014559999999999997, "Y"=56511.399999999994}, {"X"=-0.012839999999999997, "Y"=56511.399999999994}, {"X"=-0.010599999999999998, "Y"=56511.399999999994}, {"X"=-0.007960000000000002, "Y"=56511.399999999994}, {"X"=-0.00732, "Y"=56511.399999999994}, {"X"=-0.006280000000000001, "Y"=56511.399999999994}, {"X"=-0.004920000000000001, "Y"=56511.399999999994}, {"X"=-0.0046, "Y"=56511.399999999994}, {"X"=-0.047040000000000005, "Y"=58604.42000000001}, {"X"=-0.045520000000000005, "Y"=58604.42000000001}, {"X"=-0.04472, "Y"=58604.42000000001}, {"X"=-0.043320000000000004, "Y"=58604.42000000001}, {"X"=-0.04124, "Y"=58604.42000000001}, {"X"=-0.04048, "Y"=58604.42000000001}, {"X"=-0.0396, "Y"=58604.42000000001}, {"X"=-0.03848, "Y"=58604.42000000001}, {"X"=-0.037680000000000005, "Y"=58604.42000000001}, {"X"=-0.03712, "Y"=58604.42000000001}, {"X"=-0.0364, "Y"=58604.42000000001}, {"X"=-0.03484, "Y"=58604.42000000001}, {"X"=-0.03312, "Y"=58604.42000000001}, {"X"=-0.03184, "Y"=58604.42000000001}, {"X"=-0.0304, "Y"=58604.42000000001}, {"X"=-0.02852, "Y"=58604.42000000001}, {"X"=-0.027960000000000002, "Y"=58604.42000000001}, {"X"=-0.02536, "Y"=58604.42000000001}, {"X"=-0.0218, "Y"=58604.42000000001}, {"X"=-0.020640000000000002, "Y"=58604.42000000001}, {"X"=-0.0204, "Y"=58604.42000000001}, {"X"=-0.01856, "Y"=58604.42000000001}, {"X"=-0.016440000000000003, "Y"=58604.42000000001}, {"X"=-0.014559999999999997, "Y"=58604.42000000001}, {"X"=-0.012880000000000003, "Y"=58604.42000000001}, {"X"=-0.010439999999999998, "Y"=58604.42000000001}, {"X"=-0.008239999999999997, "Y"=58604.42000000001}, {"X"=-0.007199999999999998, "Y"=58604.42000000001}, {"X"=-0.004920000000000001, "Y"=58604.42000000001}, {"X"=-0.04696, "Y"=60697.44}, {"X"=-0.044520000000000004, "Y"=60697.44}, {"X"=-0.04324, "Y"=60697.44}, {"X"=-0.041080000000000005, "Y"=60697.44}, {"X"=-0.040400000000000005, "Y"=60697.44}, {"X"=-0.0396, "Y"=60697.44}, {"X"=-0.03828, "Y"=60697.44}, {"X"=-0.03784, "Y"=60697.44}, {"X"=-0.037320000000000006, "Y"=60697.44}, {"X"=-0.03628, "Y"=60697.44}, {"X"=-0.0348, "Y"=60697.44}, {"X"=-0.033, "Y"=60697.44}, {"X"=-0.03184, "Y"=60697.44}, {"X"=-0.03136, "Y"=60697.44}, {"X"=-0.030160000000000003, "Y"=60697.44}, {"X"=-0.02844, "Y"=60697.44}, {"X"=-0.02708, "Y"=60697.44}, {"X"=-0.025160000000000002, "Y"=60697.44}, {"X"=-0.02164, "Y"=60697.44}, {"X"=-0.0204, "Y"=60697.44}, {"X"=-0.018520000000000002, "Y"=60697.44}, {"X"=-0.0174, "Y"=60697.44}, {"X"=-0.016239999999999997, "Y"=60697.44}, {"X"=-0.014400000000000003, "Y"=60697.44}, {"X"=-0.012799999999999999, "Y"=60697.44}, {"X"=-0.010279999999999997, "Y"=60697.44}, {"X"=-0.008079999999999997, "Y"=60697.44}, {"X"=-0.004679999999999997, "Y"=60697.44}, {"X"=-0.04696, "Y"=62790.45999999999}, {"X"=-0.04444, "Y"=62790.45999999999}, {"X"=-0.043320000000000004, "Y"=62790.45999999999}, {"X"=-0.041, "Y"=62790.45999999999}, {"X"=-0.04052, "Y"=62790.45999999999}, {"X"=-0.03968, "Y"=62790.45999999999}, {"X"=-0.0382, "Y"=62790.45999999999}, {"X"=-0.03624, "Y"=62790.45999999999}, {"X"=-0.03484, "Y"=62790.45999999999}, {"X"=-0.033, "Y"=62790.45999999999}, {"X"=-0.031920000000000004, "Y"=62790.45999999999}, {"X"=-0.03124, "Y"=62790.45999999999}, {"X"=-0.03004, "Y"=62790.45999999999}, {"X"=-0.02844, "Y"=62790.45999999999}, {"X"=-0.02708, "Y"=62790.45999999999}, {"X"=-0.02508, "Y"=62790.45999999999}, {"X"=-0.0216, "Y"=62790.45999999999}, {"X"=-0.02068, "Y"=62790.45999999999}, {"X"=-0.0186, "Y"=62790.45999999999}, {"X"=-0.0172, "Y"=62790.45999999999}, {"X"=-0.01616, "Y"=62790.45999999999}, {"X"=-0.014879999999999997, "Y"=62790.45999999999}, {"X"=-0.01412, "Y"=62790.45999999999}, {"X"=-0.012799999999999999, "Y"=62790.45999999999}, {"X"=-0.010119999999999997, "Y"=62790.45999999999}, {"X"=-0.008120000000000002, "Y"=62790.45999999999}, {"X"=-0.006359999999999998, "Y"=62790.45999999999}, {"X"=-0.004639999999999998, "Y"=62790.45999999999}, {"X"=-0.047040000000000005, "Y"=64883.48000000001}, {"X"=-0.04444, "Y"=64883.48000000001}, {"X"=-0.0434, "Y"=64883.48000000001}, {"X"=-0.040720000000000006, "Y"=64883.48000000001}, {"X"=-0.039760000000000004, "Y"=64883.48000000001}, {"X"=-0.0382, "Y"=64883.48000000001}, {"X"=-0.03628, "Y"=64883.48000000001}, {"X"=-0.03492, "Y"=64883.48000000001}, {"X"=-0.03308, "Y"=64883.48000000001}, {"X"=-0.032, "Y"=64883.48000000001}, {"X"=-0.031200000000000002, "Y"=64883.48000000001}, {"X"=-0.030000000000000002, "Y"=64883.48000000001}, {"X"=-0.02852, "Y"=64883.48000000001}, {"X"=-0.02716, "Y"=64883.48000000001}, {"X"=-0.02508, "Y"=64883.48000000001}, {"X"=-0.02156, "Y"=64883.48000000001}, {"X"=-0.02076, "Y"=64883.48000000001}, {"X"=-0.018680000000000002, "Y"=64883.48000000001}, {"X"=-0.0172, "Y"=64883.48000000001}, {"X"=-0.015039999999999998, "Y"=64883.48000000001}, {"X"=-0.014080000000000002, "Y"=64883.48000000001}, {"X"=-0.013159999999999998, "Y"=64883.48000000001}, {"X"=-0.012880000000000003, "Y"=64883.48000000001}, {"X"=-0.01004, "Y"=64883.48000000001}, {"X"=-0.00816, "Y"=64883.48000000001}, {"X"=-0.004720000000000002, "Y"=64883.48000000001}, {"X"=-0.047040000000000005, "Y"=66976.5}, {"X"=-0.044360000000000004, "Y"=66976.5}, {"X"=-0.0434, "Y"=66976.5}, {"X"=-0.040720000000000006, "Y"=66976.5}, {"X"=-0.0398, "Y"=66976.5}, {"X"=-0.03808, "Y"=66976.5}, {"X"=-0.0368, "Y"=66976.5}, {"X"=-0.0362, "Y"=66976.5}, {"X"=-0.034960000000000005, "Y"=66976.5}, {"X"=-0.03304, "Y"=66976.5}, {"X"=-0.03204, "Y"=66976.5}, {"X"=-0.03108, "Y"=66976.5}, {"X"=-0.02988, "Y"=66976.5}, {"X"=-0.028560000000000002, "Y"=66976.5}, {"X"=-0.028120000000000003, "Y"=66976.5}, {"X"=-0.02708, "Y"=66976.5}, {"X"=-0.02504, "Y"=66976.5}, {"X"=-0.02144, "Y"=66976.5}, {"X"=-0.02072, "Y"=66976.5}, {"X"=-0.018680000000000002, "Y"=66976.5}, {"X"=-0.017079999999999998, "Y"=66976.5}, {"X"=-0.015199999999999998, "Y"=66976.5}, {"X"=-0.0138, "Y"=66976.5}, {"X"=-0.012920000000000001, "Y"=66976.5}, {"X"=-0.00988, "Y"=66976.5}, {"X"=-0.00816, "Y"=66976.5}, {"X"=-0.006999999999999999, "Y"=66976.5}, {"X"=-0.00596, "Y"=66976.5}, {"X"=-0.0045600000000000016, "Y"=66976.5}, {"X"=-0.04712, "Y"=69069.51999999999}, {"X"=-0.044320000000000005, "Y"=69069.51999999999}, {"X"=-0.043480000000000005, "Y"=69069.51999999999}, {"X"=-0.040720000000000006, "Y"=69069.51999999999}, {"X"=-0.03984, "Y"=69069.51999999999}, {"X"=-0.03812, "Y"=69069.51999999999}, {"X"=-0.03764, "Y"=69069.51999999999}, {"X"=-0.03688, "Y"=69069.51999999999}, {"X"=-0.03624, "Y"=69069.51999999999}, {"X"=-0.03504, "Y"=69069.51999999999}, {"X"=-0.03308, "Y"=69069.51999999999}, {"X"=-0.03212, "Y"=69069.51999999999}, {"X"=-0.031, "Y"=69069.51999999999}, {"X"=-0.0298, "Y"=69069.51999999999}, {"X"=-0.028640000000000002, "Y"=69069.51999999999}, {"X"=-0.0282, "Y"=69069.51999999999}, {"X"=-0.027, "Y"=69069.51999999999}, {"X"=-0.02504, "Y"=69069.51999999999}, {"X"=-0.0214, "Y"=69069.51999999999}, {"X"=-0.02076, "Y"=69069.51999999999}, {"X"=-0.01872, "Y"=69069.51999999999}, {"X"=-0.01704, "Y"=69069.51999999999}, {"X"=-0.015399999999999997, "Y"=69069.51999999999}, {"X"=-0.01364, "Y"=69069.51999999999}, {"X"=-0.012799999999999999, "Y"=69069.51999999999}, {"X"=-0.010360000000000001, "Y"=69069.51999999999}, {"X"=-0.009599999999999997, "Y"=69069.51999999999}, {"X"=-0.00816, "Y"=69069.51999999999}, {"X"=-0.006080000000000002, "Y"=69069.51999999999}, {"X"=-0.0056799999999999976, "Y"=69069.51999999999}, {"X"=-0.047080000000000004, "Y"=71162.54000000001}, {"X"=-0.04428, "Y"=71162.54000000001}, {"X"=-0.04356, "Y"=71162.54000000001}, {"X"=-0.0412, "Y"=71162.54000000001}, {"X"=-0.04068, "Y"=71162.54000000001}, {"X"=-0.03988, "Y"=71162.54000000001}, {"X"=-0.03812, "Y"=71162.54000000001}, {"X"=-0.0376, "Y"=71162.54000000001}, {"X"=-0.0366, "Y"=71162.54000000001}, {"X"=-0.03612, "Y"=71162.54000000001}, {"X"=-0.03512, "Y"=71162.54000000001}, {"X"=-0.03216, "Y"=71162.54000000001}, {"X"=-0.03092, "Y"=71162.54000000001}, {"X"=-0.028640000000000002, "Y"=71162.54000000001}, {"X"=-0.02692, "Y"=71162.54000000001}, {"X"=-0.025, "Y"=71162.54000000001}, {"X"=-0.021320000000000002, "Y"=71162.54000000001}, {"X"=-0.02068, "Y"=71162.54000000001}, {"X"=-0.018680000000000002, "Y"=71162.54000000001}, {"X"=-0.017, "Y"=71162.54000000001}, {"X"=-0.015440000000000002, "Y"=71162.54000000001}, {"X"=-0.013519999999999997, "Y"=71162.54000000001}, {"X"=-0.012839999999999997, "Y"=71162.54000000001}, {"X"=-0.010279999999999997, "Y"=71162.54000000001}, {"X"=-0.009480000000000002, "Y"=71162.54000000001}, {"X"=-0.008320000000000001, "Y"=71162.54000000001}, {"X"=-0.008039999999999999, "Y"=71162.54000000001}, {"X"=-0.005719999999999996, "Y"=71162.54000000001}, {"X"=-0.047080000000000004, "Y"=73255.56}, {"X"=-0.0446, "Y"=73255.56}, {"X"=-0.04372, "Y"=73255.56}, {"X"=-0.04148, "Y"=73255.56}, {"X"=-0.040720000000000006, "Y"=73255.56}, {"X"=-0.040040000000000006, "Y"=73255.56}, {"X"=-0.03816, "Y"=73255.56}, {"X"=-0.03616, "Y"=73255.56}, {"X"=-0.03512, "Y"=73255.56}, {"X"=-0.03388, "Y"=73255.56}, {"X"=-0.03216, "Y"=73255.56}, {"X"=-0.0308, "Y"=73255.56}, {"X"=-0.02892, "Y"=73255.56}, {"X"=-0.02732, "Y"=73255.56}, {"X"=-0.026520000000000002, "Y"=73255.56}, {"X"=-0.025160000000000002, "Y"=73255.56}, {"X"=-0.021320000000000002, "Y"=73255.56}, {"X"=-0.02052, "Y"=73255.56}, {"X"=-0.01872, "Y"=73255.56}, {"X"=-0.016919999999999998, "Y"=73255.56}, {"X"=-0.01532, "Y"=73255.56}, {"X"=-0.013400000000000002, "Y"=73255.56}, {"X"=-0.012839999999999997, "Y"=73255.56}, {"X"=-0.010119999999999997, "Y"=73255.56}, {"X"=-0.009279999999999997, "Y"=73255.56}, {"X"=-0.008079999999999997, "Y"=73255.56}, {"X"=-0.005760000000000001, "Y"=73255.56}, {"X"=-0.005159999999999998, "Y"=73255.56}, {"X"=-0.0046, "Y"=73255.56}, {"X"=-0.04744, "Y"=75348.57999999999}, {"X"=-0.0444, "Y"=75348.57999999999}, {"X"=-0.043800000000000006, "Y"=75348.57999999999}, {"X"=-0.041280000000000004, "Y"=75348.57999999999}, {"X"=-0.04064, "Y"=75348.57999999999}, {"X"=-0.040040000000000006, "Y"=75348.57999999999}, {"X"=-0.03824, "Y"=75348.57999999999}, {"X"=-0.03644, "Y"=75348.57999999999}, {"X"=-0.035320000000000004, "Y"=75348.57999999999}, {"X"=-0.0324, "Y"=75348.57999999999}, {"X"=-0.03092, "Y"=75348.57999999999}, {"X"=-0.02884, "Y"=75348.57999999999}, {"X"=-0.02768, "Y"=75348.57999999999}, {"X"=-0.02684, "Y"=75348.57999999999}, {"X"=-0.02488, "Y"=75348.57999999999}, {"X"=-0.022520000000000002, "Y"=75348.57999999999}, {"X"=-0.02164, "Y"=75348.57999999999}, {"X"=-0.02088, "Y"=75348.57999999999}, {"X"=-0.01908, "Y"=75348.57999999999}, {"X"=-0.01716, "Y"=75348.57999999999}, {"X"=-0.01564, "Y"=75348.57999999999}, {"X"=-0.013839999999999998, "Y"=75348.57999999999}, {"X"=-0.013319999999999999, "Y"=75348.57999999999}, {"X"=-0.012799999999999999, "Y"=75348.57999999999}, {"X"=-0.010439999999999998, "Y"=75348.57999999999}, {"X"=-0.009439999999999997, "Y"=75348.57999999999}, {"X"=-0.008399999999999998, "Y"=75348.57999999999}, {"X"=-0.006039999999999997, "Y"=75348.57999999999}, {"X"=-0.004720000000000002, "Y"=75348.57999999999}, {"X"=-0.04736, "Y"=77441.6}, {"X"=-0.04428, "Y"=77441.6}, {"X"=-0.04372, "Y"=77441.6}, {"X"=-0.042120000000000005, "Y"=77441.6}, {"X"=-0.04116, "Y"=77441.6}, {"X"=-0.04048, "Y"=77441.6}, {"X"=-0.03996, "Y"=77441.6}, {"X"=-0.03808, "Y"=77441.6}, {"X"=-0.0364, "Y"=77441.6}, {"X"=-0.036000000000000004, "Y"=77441.6}, {"X"=-0.03524, "Y"=77441.6}, {"X"=-0.03236, "Y"=77441.6}, {"X"=-0.0308, "Y"=77441.6}, {"X"=-0.02888, "Y"=77441.6}, {"X"=-0.026760000000000003, "Y"=77441.6}, {"X"=-0.02552, "Y"=77441.6}, {"X"=-0.02476, "Y"=77441.6}, {"X"=-0.022600000000000002, "Y"=77441.6}, {"X"=-0.02144, "Y"=77441.6}, {"X"=-0.02084, "Y"=77441.6}, {"X"=-0.01912, "Y"=77441.6}, {"X"=-0.01704, "Y"=77441.6}, {"X"=-0.015760000000000003, "Y"=77441.6}, {"X"=-0.013479999999999999, "Y"=77441.6}, {"X"=-0.009439999999999997, "Y"=77441.6}, {"X"=-0.009079999999999998, "Y"=77441.6}, {"X"=-0.008280000000000003, "Y"=77441.6}, {"X"=-0.006159999999999999, "Y"=77441.6}, {"X"=-0.005639999999999999, "Y"=77441.6}, {"X"=-0.047560000000000005, "Y"=79534.62}, {"X"=-0.0444, "Y"=79534.62}, {"X"=-0.04392, "Y"=79534.62}, {"X"=-0.04232, "Y"=79534.62}, {"X"=-0.04136, "Y"=79534.62}, {"X"=-0.04048, "Y"=79534.62}, {"X"=-0.04016, "Y"=79534.62}, {"X"=-0.03816, "Y"=79534.62}, {"X"=-0.0366, "Y"=79534.62}, {"X"=-0.03612, "Y"=79534.62}, {"X"=-0.035320000000000004, "Y"=79534.62}, {"X"=-0.03248, "Y"=79534.62}, {"X"=-0.030760000000000003, "Y"=79534.62}, {"X"=-0.029, "Y"=79534.62}, {"X"=-0.028040000000000002, "Y"=79534.62}, {"X"=-0.026680000000000002, "Y"=79534.62}, {"X"=-0.02556, "Y"=79534.62}, {"X"=-0.0246, "Y"=79534.62}, {"X"=-0.02224, "Y"=79534.62}, {"X"=-0.02164, "Y"=79534.62}, {"X"=-0.02072, "Y"=79534.62}, {"X"=-0.01916, "Y"=79534.62}, {"X"=-0.017, "Y"=79534.62}, {"X"=-0.015919999999999997, "Y"=79534.62}, {"X"=-0.013560000000000003, "Y"=79534.62}, {"X"=-0.012920000000000001, "Y"=79534.62}, {"X"=-0.010279999999999997, "Y"=79534.62}, {"X"=-0.009279999999999997, "Y"=79534.62}, {"X"=-0.0061200000000000004, "Y"=79534.62}, {"X"=-0.04764, "Y"=81627.63999999998}, {"X"=-0.04444, "Y"=81627.63999999998}, {"X"=-0.04396, "Y"=81627.63999999998}, {"X"=-0.0424, "Y"=81627.63999999998}, {"X"=-0.04132, "Y"=81627.63999999998}, {"X"=-0.04032, "Y"=81627.63999999998}, {"X"=-0.03812, "Y"=81627.63999999998}, {"X"=-0.036320000000000005, "Y"=81627.63999999998}, {"X"=-0.035840000000000004, "Y"=81627.63999999998}, {"X"=-0.03536, "Y"=81627.63999999998}, {"X"=-0.03248, "Y"=81627.63999999998}, {"X"=-0.030680000000000002, "Y"=81627.63999999998}, {"X"=-0.02908, "Y"=81627.63999999998}, {"X"=-0.028, "Y"=81627.63999999998}, {"X"=-0.02664, "Y"=81627.63999999998}, {"X"=-0.02564, "Y"=81627.63999999998}, {"X"=-0.024480000000000002, "Y"=81627.63999999998}, {"X"=-0.022520000000000002, "Y"=81627.63999999998}, {"X"=-0.02208, "Y"=81627.63999999998}, {"X"=-0.020640000000000002, "Y"=81627.63999999998}, {"X"=-0.01924, "Y"=81627.63999999998}, {"X"=-0.016800000000000002, "Y"=81627.63999999998}, {"X"=-0.01604, "Y"=81627.63999999998}, {"X"=-0.013600000000000001, "Y"=81627.63999999998}, {"X"=-0.01276, "Y"=81627.63999999998}, {"X"=-0.011279999999999998, "Y"=81627.63999999998}, {"X"=-0.010160000000000002, "Y"=81627.63999999998}, {"X"=-0.009239999999999998, "Y"=81627.63999999998}, {"X"=-0.008919999999999997, "Y"=81627.63999999998}, {"X"=-0.007879999999999998, "Y"=81627.63999999998}, {"X"=-0.006319999999999999, "Y"=81627.63999999998}, {"X"=-0.04764, "Y"=83720.66}, {"X"=-0.04444, "Y"=83720.66}, {"X"=-0.04388, "Y"=83720.66}, {"X"=-0.042480000000000004, "Y"=83720.66}, {"X"=-0.04132, "Y"=83720.66}, {"X"=-0.04028, "Y"=83720.66}, {"X"=-0.03808, "Y"=83720.66}, {"X"=-0.03548, "Y"=83720.66}, {"X"=-0.03252, "Y"=83720.66}, {"X"=-0.03056, "Y"=83720.66}, {"X"=-0.02912, "Y"=83720.66}, {"X"=-0.02552, "Y"=83720.66}, {"X"=-0.02432, "Y"=83720.66}, {"X"=-0.02236, "Y"=83720.66}, {"X"=-0.02156, "Y"=83720.66}, {"X"=-0.02048, "Y"=83720.66}, {"X"=-0.01916, "Y"=83720.66}, {"X"=-0.016599999999999997, "Y"=83720.66}, {"X"=-0.01344, "Y"=83720.66}, {"X"=-0.012679999999999997, "Y"=83720.66}, {"X"=-0.01124, "Y"=83720.66}, {"X"=-0.009919999999999998, "Y"=83720.66}, {"X"=-0.009480000000000002, "Y"=83720.66}, {"X"=-0.008599999999999997, "Y"=83720.66}, {"X"=-0.006080000000000002, "Y"=83720.66}, {"X"=-0.0476, "Y"=85813.68}, {"X"=-0.0444, "Y"=85813.68}, {"X"=-0.04376, "Y"=85813.68}, {"X"=-0.042480000000000004, "Y"=85813.68}, {"X"=-0.041280000000000004, "Y"=85813.68}, {"X"=-0.04016, "Y"=85813.68}, {"X"=-0.038000000000000006, "Y"=85813.68}, {"X"=-0.03724, "Y"=85813.68}, {"X"=-0.036000000000000004, "Y"=85813.68}, {"X"=-0.035320000000000004, "Y"=85813.68}, {"X"=-0.03252, "Y"=85813.68}, {"X"=-0.0304, "Y"=85813.68}, {"X"=-0.029160000000000002, "Y"=85813.68}, {"X"=-0.02816, "Y"=85813.68}, {"X"=-0.02548, "Y"=85813.68}, {"X"=-0.02412, "Y"=85813.68}, {"X"=-0.02236, "Y"=85813.68}, {"X"=-0.0216, "Y"=85813.68}, {"X"=-0.0204, "Y"=85813.68}, {"X"=-0.019200000000000002, "Y"=85813.68}, {"X"=-0.0162, "Y"=85813.68}, {"X"=-0.013400000000000002, "Y"=85813.68}, {"X"=-0.012240000000000001, "Y"=85813.68}, {"X"=-0.009640000000000003, "Y"=85813.68}, {"X"=-0.008559999999999998, "Y"=85813.68}, {"X"=-0.007679999999999999, "Y"=85813.68}, {"X"=-0.005080000000000001, "Y"=85813.68}]
  out "Vsg vs B":cluster{"X":dbl, "Y":dbl}[](graph)
  in  "stop":bool
  in  "Vsg vs B 2":cluster{"X":dbl, "Y":dbl}[](graph)
  in  "Coupling factor (eV/V)":dbl=0.1
  out "Bc":cluster{"Bc+":dbl, "Bc-":dbl, "Bc ave":dbl}={"Bc+"=nan, "Bc-"=nan, "Bc ave"=nan}
  out "g factor":cluster{"g+":dbl, "g-":dbl, "g ave":dbl}={"g+"=nan, "g-"=nan, "g ave"=nan}
  out "Bc error":T1={"Bc+ error (Oe)"=nan, "Bc- error (Oe)"=nan, "Bc error ave"=nan}
  in  "Coupling factor error":dbl
  out "g factor error":T2={"g+ error"=nan, "g- error"=nan, "g error"=nan}
  out "XY Graph 6":cluster{dbl[], dbl[]}[](graph)
  in  "OK Button 2":bool
  out "Vsg":dbl=-0.005400000000000002
  in  "page one":bool
  in  "Write to ITX":bool
  in  "saved ITX":path=path "P:/expt/IQC/2011-summer Superconductivity-Spin Hall/Data/SA02670K.20130810/Processed Data/Bc vs Vsg"
  in  "filename":string="manual_splitting"
  in  "Comment":string="SA02670K.20130810\nPD threshold -6 "
  in  "stop 2":bool
  in  "page one 2":bool
  out "2D Error Bar":refnum<class "2D Plot Datatype.lvclass">[](xcontrol)
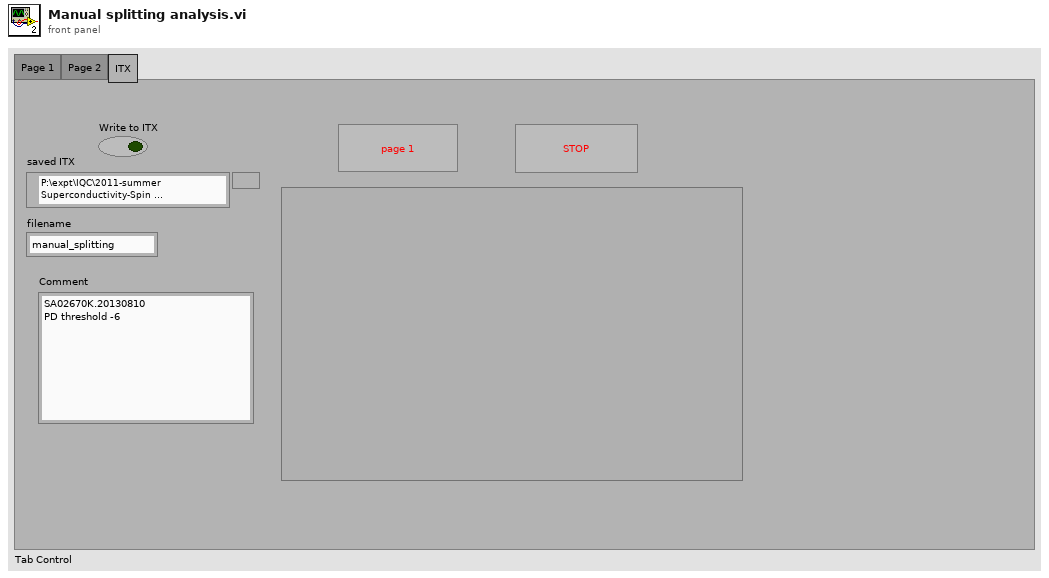
[diagram p1: front panel]
types:
  T1 = cluster{"Bc+ error (Oe)":dbl, "Bc- error (Oe)":dbl, "Bc error ave":dbl}
  T2 = cluster{"g+ error":dbl, "g- error":dbl, "g error":dbl}
  T3 = cluster{"sigma_A (Oe)":dbl, "sigma_A (Oe)":dbl, dbl}
  T4 = cluster{"sigma_A (Oe)":dbl, "sigma_A (Oe)":dbl, dbl}[]
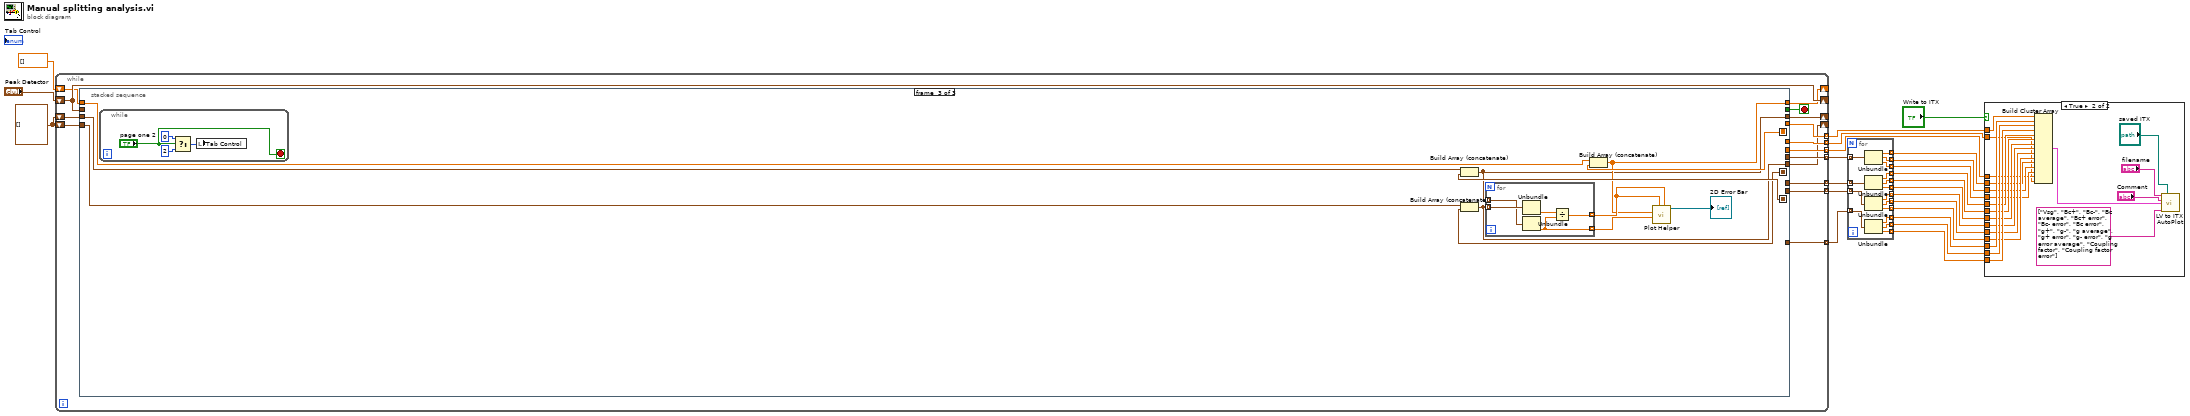
[diagram p0: block diagram]
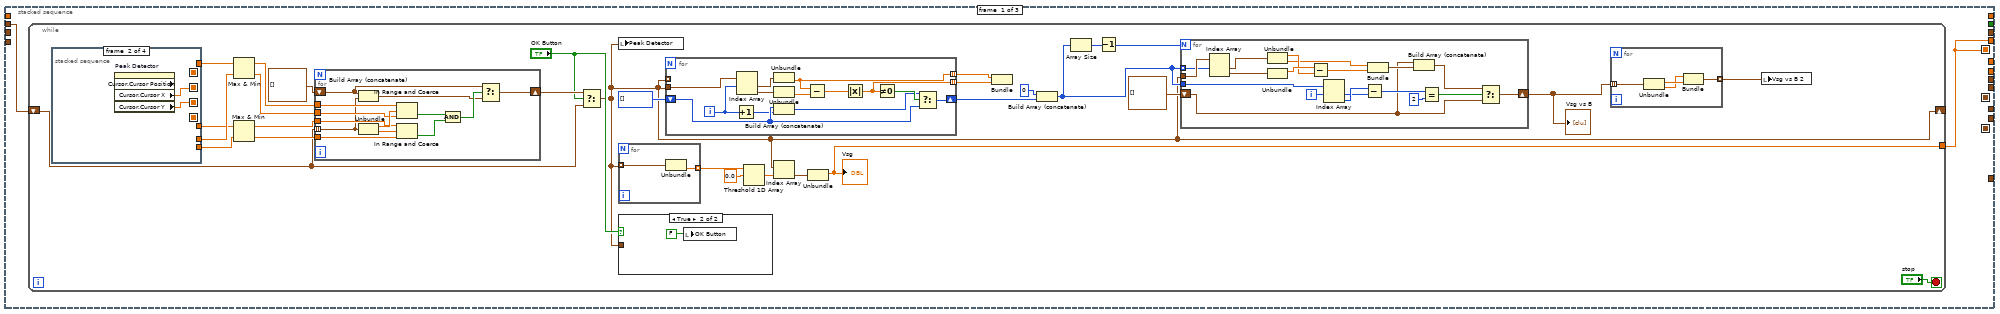
[diagram p3: hidden frame]
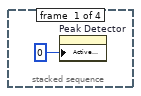
[diagram p5: hidden frame]
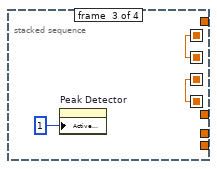
[diagram p6: hidden frame]
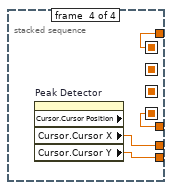
[diagram p7: hidden frame]
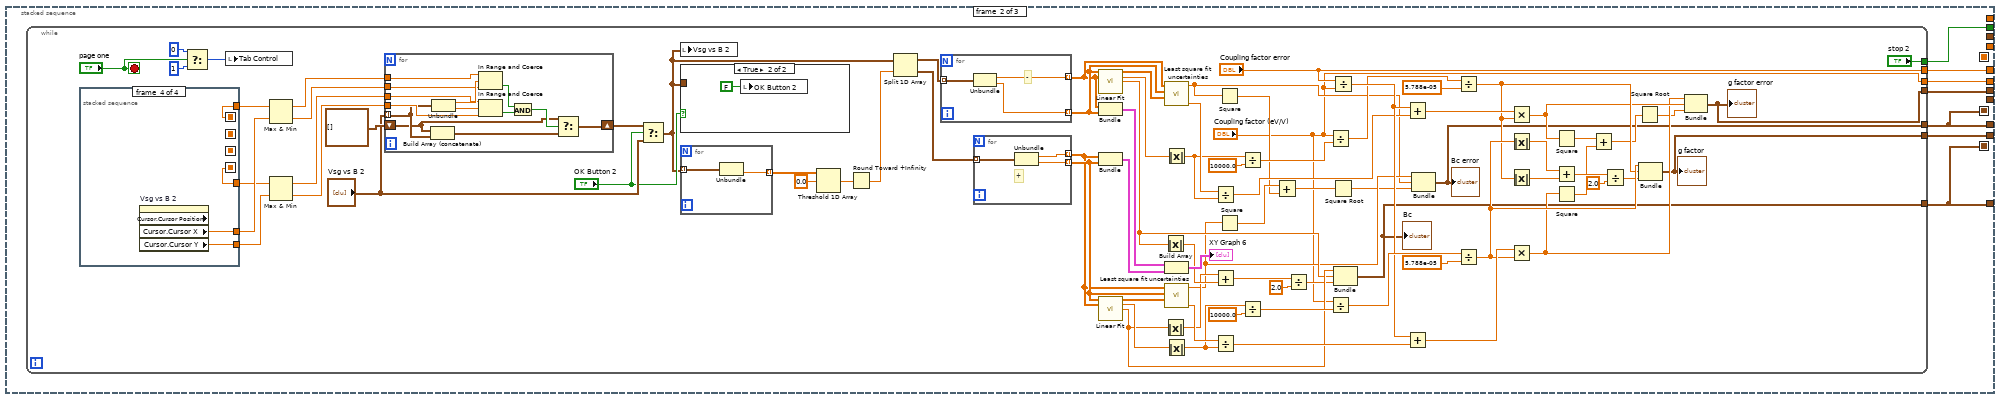
[diagram p8: hidden frame]
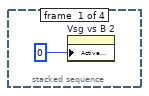
[diagram p10: hidden frame]
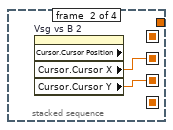
[diagram p11: hidden frame]
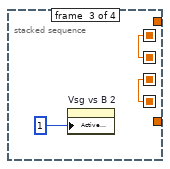
[diagram p12: hidden frame]
diagram:
  w1 = cluster{"intercept":dbl, "intercept":dbl, dbl}[] []
  n1 = while {
    tunnel: [w30] -> w23 mode=indexing
    tunnel: [w38] -> w22 mode=indexing
    tunnel: [w37] -> w21 mode=indexing
    tunnel: [w36] -> w20 mode=indexing
    tunnel: [w29] -> w19 mode=indexing
    tunnel: [w35] -> w5 mode=indexing
    tunnel: [w34] -> w6 mode=indexing
    shift-right: [w32] -> _
    shift-left: "Peak Detector" -> [w32]
    shift-right: [w25] -> _
    shift-left: w1 -> [w31]
    shift-right: [w26] -> _
    shift-left: dbl[] [] -> [w28]
    shift-right: [w24] -> _
    shift-left: w1 -> [w27]
    stop <- w33 stop-if-true
    n2 = stacked-sequence {
      seq-local: [w39 _ _] -> [_ _ w264]
      seq-local: [_ w134 _] -> [_ _ w261]
      seq-local: [_ w133 _] -> [_ _ w258]
      tunnel: [_ w134 _] -> w30
      tunnel: [_ w133 _] -> w38
      tunnel: [_ w139 _] -> w36
      tunnel: [_ w138 _] -> w37
      tunnel: w32 -> [w40 _ _]
      tunnel: [w39 _ _] -> w29
      tunnel: [_ w137 _] -> w35
      tunnel: [_ w136 _] -> w34
      tunnel: [_ w135 _] -> w33
      tunnel: w31 -> [_ _ w262]
      tunnel: w28 -> [_ _ w263]
      tunnel: w27 -> [_ _ w259]
      tunnel: [_ _ w260] -> w26
      tunnel: [_ _ w256] -> w25
      tunnel: [_ _ w257] -> w24
      frame #0 {
        n3 = while {
          shift-right: [w43] -> _
          shift-left: w40 -> [w45]
          tunnel: [w44] -> w39
          stop <- "stop" stop-if-true
          n4 = stacked-sequence {
            seq-local: [_ w76 _ _] -> [_ _ w78 _]
            seq-local: [_ w75 _ _] -> [_ _ w77 _]
            seq-local: [_ _ w78 _] -> [_ _ _ w83]
            seq-local: [_ _ w77 _] -> [_ _ _ w81]
            tunnel: [_ _ _ w83] -> w70
            tunnel: [_ _ _ w82] -> w69
            tunnel: [_ _ _ w81] -> w68
            tunnel: [_ _ _ w80] -> w67
            frame #0 {
              n5 = property on="Peak Detector" class="XYGraph (strict)"("Active Cursor"=u32 0) -> ()  [unwired: 2 in, 2 out]
            }
            frame #1 {
              n6 = property on="Peak Detector" class="XYGraph (strict)" props=["Cursor", "Cursor Position", "Cursor", "Cursor X", "Cursor", "Cursor Y"]() -> ("Cursor.Cursor X"=w76:dbl, "Cursor.Cursor Y"=w75:dbl)  [unwired: 2 in, 3 out]
            }
            frame #2 {
              n7 = property on="Peak Detector" class="XYGraph (strict)"("Active Cursor"=u32 1) -> ()  [unwired: 2 in, 2 out]
            }
            frame #3 {
              n8 = property on="Peak Detector" class="XYGraph (strict)" props=["Cursor", "Cursor Position", "Cursor", "Cursor X", "Cursor", "Cursor Y"]() -> ("Cursor.Cursor X"=w82:dbl, "Cursor.Cursor Y"=w80:dbl)  [unwired: 2 in, 3 out]
            }
          }
          n9 = Max & Min(x=w70, y=w69) -> (max(x,y)=w66:dbl, min(x,y)=w65:dbl)
          n10 = Max & Min(x=w68, y=w67) -> (max(x,y)=w64:dbl, min(x,y)=w63:dbl)
          n11 = for {
            tunnel: w45 -> [w119] mode=indexing
            tunnel: w66 -> [w127]
            tunnel: w65 -> [w126]
            tunnel: w64 -> [w124]
            tunnel: w63 -> [w123]
            shift-right: [w118] -> w54
            shift-left: cluster{"X":dbl, "Y":dbl}[] [] -> [w117]
            n12 = Build Array (concatenate)(w117, w119) -> (w116:cluster{"X":dbl, "Y":dbl}[])
            n13 = Unbundle(w119) -> ("X"=w128:dbl, "Y"=w125:dbl)
            n14 = In Range and Coerce(upper limit=w127, x=w128, lower limit=w126) -> (In Range?=w122:bool)  [unwired: 1 out]
            n15 = In Range and Coerce(upper limit=w124, x=w125, lower limit=w123) -> (In Range?=w121:bool)  [unwired: 1 out]
            n16 = And(x=w122, y=w121) -> (x .and. y?=w120:bool)
            n17 = Select(t=w117, s=w120, f=w116) -> (s? t:f=w118:cluster{"X":dbl, "Y":dbl}[])
          }
          n18 = Select(t=w54, s="OK Button", f=w45) -> (s? t:f=w43:cluster{"X":dbl, "Y":dbl}[])
          n19 = local write "Peak Detector"(w43) -> ()
          n20 = for {
            tunnel: w43 -> [w72] mode=indexing
            tunnel: [w71] -> w49 mode=indexing
            n21 = Unbundle(w72) -> ("Y"=w71:dbl)  [unwired: 1 out]
          }
          n22 = case shown="True" "OK Button" {
            tunnel: w43 -> [_ _]
            frame False {
            }
            frame True {
              n23 = local write "OK Button"(FALSE ("OK Button")) -> ()
            }
          }
          n24 = for {
            tunnel: w43 -> [w115]
            tunnel: w43 -> [_] mode=indexing
            shift-right: [w107] -> w59
            shift-left: i32[] [] -> [w106]
            tunnel: [w104] -> w41 mode=indexing
            tunnel: [w103] -> w42 mode=indexing
            i -> [w109]
            n25 = Increment(x=w109) -> (x+1=w105:i32)
            n26 = Index Array(array=w115, index #1=w109) -> (element #1=w114:cluster{"X":dbl, "Y":dbl}, element #2=w113:cluster{"X":dbl, "Y":dbl})  [unwired: 1 in]
            n27 = Unbundle(w114) -> ("Y"=w103:dbl)  [unwired: 1 out]
            n28 = Unbundle(w113) -> ("Y"=w112:dbl)  [unwired: 1 out]
            n29 = Build Array (concatenate)(w106, w105) -> (w108:i32[])
            n30 = Subtract(x=w103, y=w112) -> (x-y=w111:dbl)
            n31 = Absolute Value(x=w111) -> (abs(x)=w104:dbl)
            n32 = Not Equal To 0?(x=w104) -> (x != 0?=w110:bool)
            n33 = Select(t=w108, s=w110, f=w106) -> (s? t:f=w107:i32[])
          }
          n34 = Threshold 1D Array(2:0.0 ("threshold y"), 3:w49) -> (0:w47:dbl)  [unwired: 1 in]
          n35 = Index Array(array=w43, index=w47) -> (element=w50:cluster{"X":dbl, "Y":dbl})
          n36 = Unbundle(w50) -> ("X"=w44:dbl)  [unwired: 1 out]
          "Vsg" <- w44
          n37 = Bundle(w42, w41) -> ()  [unwired: 1 in, 1 out]
          n38 = Build Array (concatenate)(0, w59) -> (w56:i32[])
          n39 = Array Size(array=w56) -> (size(s)=w58:i32)
          n40 = Decrement(x=w58) -> (x-1=w57:i32)
          n41 = for {
            N: w57 -> [_]
            tunnel: w56 -> [w102]
            tunnel: w43 -> [w96]
            tunnel: w56 -> [w95] mode=indexing
            shift-right: [w85] -> w53
            shift-left: cluster{"Y":dbl, dbl}[] [] -> [w84]
            i -> [w101]
            n42 = Index Array(array=w96, index #1=w95) -> (element #1=w94:cluster{"X":dbl, "Y":dbl}, element #2=w93:cluster{"X":dbl, "Y":dbl})  [unwired: 1 in]
            n43 = Unbundle(w94) -> ("X"=w91:dbl, "Y"=w89:dbl)
            n44 = Unbundle(w93) -> ("X"=w92:dbl)  [unwired: 1 out]
            n45 = Subtract(x=w92, y=w91) -> (x-y=w90:dbl)
            n46 = Index Array(array=w102, index #1=w101) -> (element #1=w99:i32, element #2=w100:i32)  [unwired: 1 in]
            n47 = Subtract(x=w100, y=w99) -> (x-y=w98:i32)
            n48 = Bundle("Y"=w89, w90) -> (w87:cluster{"Y":dbl, dbl})  [unwired: 1 in]
            n49 = Build Array (concatenate)(w84, w87) -> (w86:cluster{"Y":dbl, dbl}[])
            n50 = Equal?(x=w98, y=2) -> (x = y?=w88:bool)
            n51 = Select(t=w86, s=w88, f=w84) -> (s? t:f=w85:cluster{"Y":dbl, dbl}[])
          }
          "Vsg vs B" <- w53
          n52 = for {
            tunnel: w53 -> [w132] mode=indexing
            tunnel: [w129] -> w52 mode=indexing
            n53 = Unbundle(w132) -> ("Y"=w131:dbl, w130:dbl)
            n54 = Bundle(w130, "Y"=w131) -> (w129:cluster{dbl, "Y":dbl})  [unwired: 1 in]
          }
          n55 = local write "Vsg vs B 2"(w52) -> ()
        }
      }
      frame #1 {
        n56 = while {
          tunnel: [w148] -> w134
          tunnel: [w140] -> w133
          tunnel: [w150] -> w139
          tunnel: [w149] -> w138
          tunnel: ["Coupling factor error"] -> w137
          tunnel: ["Coupling factor (eV/V)"] -> w136
          tunnel: ["stop 2"] -> w135
          stop <- "page one" stop-if-true
          n57 = stacked-sequence {
            seq-local: [_ w227 _ _] -> [_ _ w230 _]
            seq-local: [_ w226 _ _] -> [_ _ w229 _]
            seq-local: [_ _ w230 _] -> [_ _ _ w234]
            seq-local: [_ _ w229 _] -> [_ _ _ w233]
            tunnel: [_ _ _ w234] -> w193
            tunnel: [_ _ _ w232] -> w192
            tunnel: [_ _ _ w233] -> w191
            tunnel: [_ _ _ w231] -> w190
            frame #0 {
              n58 = property on="Vsg vs B 2" class="XYGraph (strict)"("Active Cursor"=u32 0) -> ()  [unwired: 2 in, 2 out]
            }
            frame #1 {
              n59 = property on="Vsg vs B 2" class="XYGraph (strict)" props=["Cursor", "Cursor Position", "Cursor", "Cursor X", "Cursor", "Cursor Y"]() -> ("Cursor.Cursor X"=w227:dbl, "Cursor.Cursor Y"=w226:dbl)  [unwired: 2 in, 3 out]
            }
            frame #2 {
              n60 = property on="Vsg vs B 2" class="XYGraph (strict)"("Active Cursor"=u32 1) -> ()  [unwired: 2 in, 2 out]
            }
            frame #3 {
              n61 = property on="Vsg vs B 2" class="XYGraph (strict)" props=["Cursor", "Cursor Position", "Cursor", "Cursor X", "Cursor", "Cursor Y"]() -> ("Cursor.Cursor X"=w232:dbl, "Cursor.Cursor Y"=w231:dbl)  [unwired: 2 in, 3 out]
            }
          }
          n62 = Select(t=0, s="page one", f=1) -> (s? t:f=w141:i32)
          n63 = local write "Tab Control"(w141) -> ()
          n64 = Max & Min(x=w193, y=w192) -> (max(x,y)=w189:dbl, min(x,y)=w188:dbl)
          n65 = Max & Min(x=w191, y=w190) -> (max(x,y)=w187:dbl, min(x,y)=w186:dbl)
          n66 = for {
            tunnel: "Vsg vs B 2" -> [w238] mode=indexing
            tunnel: w189 -> [w246]
            tunnel: w188 -> [w245]
            tunnel: w187 -> [w243]
            tunnel: w186 -> [w242]
            shift-right: [w237] -> w183
            shift-left: cluster{"X":dbl, "Y":dbl}[] [] -> [w236]
            n67 = Build Array (concatenate)(w236, w238) -> (w235:cluster{"X":dbl, "Y":dbl}[])
            n68 = Unbundle(w238) -> ("X"=w247:dbl, "Y"=w244:dbl)
            n69 = In Range and Coerce(upper limit=w246, x=w247, lower limit=w245) -> (In Range?=w241:bool)  [unwired: 1 out]
            n70 = In Range and Coerce(upper limit=w243, x=w244, lower limit=w242) -> (In Range?=w240:bool)  [unwired: 1 out]
            n71 = And(x=w241, y=w240) -> (x .and. y?=w239:bool)
            n72 = Select(t=w236, s=w239, f=w235) -> (s? t:f=w237:cluster{"X":dbl, "Y":dbl}[])
          }
          n73 = Select(t=w183, s="OK Button 2", f="Vsg vs B 2") -> (s? t:f=w179:cluster{"X":dbl, "Y":dbl}[])
          n74 = local write "Vsg vs B 2"(w179) -> ()
          n75 = case shown="True" "OK Button 2" {
            tunnel: w179 -> [_ _]
            frame False {
            }
            frame True {
              n76 = local write "OK Button 2"(FALSE ("OK Button")) -> ()
            }
          }
          n77 = for {
            tunnel: w179 -> [w255] mode=indexing
            tunnel: [w254] -> w223 mode=indexing
            n78 = Unbundle(w255) -> ("Y"=w254:dbl)  [unwired: 1 out]
          }
          n79 = Threshold 1D Array(2:0.0 ("threshold y"), 3:w223) -> (0:w177:dbl)  [unwired: 1 in]
          n80 = Round Toward +Infinity(x=w177) -> (ceil(x): smallest int >= x=w178:dbl)
          n81 = Split 1D Array(array=w179, index=w178) -> (first subarray=w182:cluster{"X":dbl, "Y":dbl}[], second subarray=w181:cluster{"X":dbl, "Y":dbl}[])
          n82 = for {
            tunnel: w182 -> [w253] mode=indexing
            tunnel: [w252] -> w210 mode=indexing
            tunnel: [w251] -> w211 mode=indexing
            # "-"
            n83 = Unbundle(w253) -> ("X"=w252:dbl, "Y"=w251:dbl)
          }
          n84 = for {
            tunnel: w181 -> [w250] mode=indexing
            tunnel: [w249] -> w207 mode=indexing
            tunnel: [w248] -> w208 mode=indexing
            # "+"
            n85 = Unbundle(w250) -> ("X"=w249:dbl, "Y"=w248:dbl)
          }
          n86 = call <vilib>:"Linear Fit.vi"("Y"=w211, "X"=w210) -> ("Best Linear Fit"=w209:dbl[], "slope"=w218:dbl, "intercept"=w174:dbl)  [unwired: 9 in, 2 out]
          n87 = Bundle(w210, w211) -> (w221:cluster{dbl[], dbl[]})  [unwired: 1 in]
          n88 = Bundle(w207, w208) -> (w220:cluster{dbl[], dbl[]})  [unwired: 1 in]
          n89 = call <vilib>:"Linear Fit.vi"("Y"=w208, "X"=w207) -> ("Best Linear Fit"=w206:dbl[], "slope"=w212:dbl, "intercept"=w176:dbl)  [unwired: 9 in, 2 out]
          n90 = Absolute Value(x=w174) -> (abs(x)=w175:dbl)
          n91 = Absolute Value(x=w176) -> (abs(x)=w173:dbl)
          n92 = call <userlib>:"Least square fit uncertainties.vi"("Best Linear Fit"=w209, "Y"=w211, "X"=w210) -> ("sigma_B (Oe/V)"=w199:dbl, "sigma_A (Oe)"=w168:dbl)  [unwired: 7 in]
          n93 = Absolute Value(x=w218) -> (abs(x)=w198:dbl)
          n94 = Build Array(w221, w220) -> (→"XY Graph 6":cluster{dbl[], dbl[]}[])
          n95 = call <userlib>:"Least square fit uncertainties.vi"("Best Linear Fit"=w206, "Y"=w208, "X"=w207) -> ("sigma_B (Oe/V)"=w203:dbl, "sigma_A (Oe)"=w169:dbl)  [unwired: 7 in]
          n96 = Absolute Value(x=w212) -> (abs(x)=w202:dbl)
          n97 = Divide(x=w199, y=w198) -> (x/y=w197:dbl)
          n98 = Add(x=w173, y=w175) -> (x+y=w172:dbl)
          n99 = Divide(x=w203, y=w202) -> (x/y=w201:dbl)
          n100 = Square(x=w168) -> (x^2=w166:dbl)
          n101 = Square(x=w169) -> (x^2=w167:dbl)
          n102 = Divide(x=w198, y=10000.0) -> (x/y=w216:dbl)
          n103 = Divide(x=w202, y=10000.0) -> (x/y=w205:dbl)
          n104 = Add(x=w167, y=w166) -> (x+y=w165:dbl)
          n105 = Divide(x=w172, y=2.0) -> (x/y=w170:dbl)
          n106 = Divide(x="Coupling factor (eV/V)", y=w216) -> (x/y=w195:dbl)
          n107 = Divide(x="Coupling factor (eV/V)", y=w205) -> (x/y=w213:dbl)
          n108 = Divide(x="Coupling factor error", y="Coupling factor (eV/V)") -> (x/y=w200:dbl)
          n109 = Square Root(x=w165) -> (sqrt(x)=w164:dbl)
          n110 = Bundle("intercept"=w176, "intercept"=w174, w170) -> (w148:cluster{"intercept":dbl, "intercept":dbl, dbl})  [unwired: 1 in]
          "Bc" <- w148
          n111 = Add(x=w200, y=w197) -> (x+y=w196:dbl)
          n112 = Add(x=w200, y=w201) -> (x+y=w194:dbl)
          n113 = Bundle("sigma_A (Oe)"=w169, "sigma_A (Oe)"=w168, w164) -> (w140:T3)  [unwired: 1 in]
          "Bc error" <- w140
          n114 = Divide(x=w195, y=5.788e-05) -> (x/y=w158:dbl)
          n115 = Divide(x=w213, y=5.788e-05) -> (x/y=w159:dbl)
          n116 = Multiply(x=w196, y=w158) -> (x*y=w153:dbl)
          n117 = Absolute Value(x=w159) -> (abs(x)=w162:dbl)
          n118 = Absolute Value(x=w158) -> (abs(x)=w163:dbl)
          n119 = Multiply(x=w194, y=w159) -> (x*y=w152:dbl)
          n120 = Square(x=w153) -> (x^2=w154:dbl)
          n121 = Add(x=w162, y=w163) -> (x+y=w161:dbl)
          n122 = Square(x=w152) -> (x^2=w155:dbl)
          n123 = Add(x=w154, y=w155) -> (x+y=w156:dbl)
          n124 = Divide(x=w161, y=2.0) -> (x/y=w157:dbl)
          n125 = Square Root(x=w156) -> (sqrt(x)=w151:dbl)
          n126 = Bundle(w159, w158, w157) -> (w149:cluster{dbl, dbl, dbl})  [unwired: 1 in]
          "g factor" <- w149
          n127 = Bundle(w152, w153, w151) -> (w150:cluster{dbl, dbl, dbl})  [unwired: 1 in]
          "g factor error" <- w150
        }
      }
      frame #2 {
        n128 = while {
          stop <- "page one 2" stop-if-true
          n129 = Select(t=0, s="page one 2", f=2) -> (s? t:f=w269:i32)
          n130 = local write "Tab Control"(w269) -> ()
        }
        n131 = Build Array (concatenate)(w262, w261) -> (w256:cluster{"intercept":dbl, "intercept":dbl, dbl}[])
        n132 = Build Array (concatenate)(w259, w258) -> (w257:T4)
        n133 = for {
          tunnel: w256 -> [w275] mode=indexing
          tunnel: w257 -> [w276] mode=indexing
          tunnel: [w273] -> w265 mode=indexing
          tunnel: [w272] -> w266 mode=indexing
          n134 = Unbundle(w276) -> (w274:dbl)  [unwired: 2 out]
          n135 = Unbundle(w275) -> (w272:dbl)  [unwired: 2 out]
          n136 = Divide(x=w274, y=w272) -> (x/y=w273:dbl)
        }
        n137 = Build Array (concatenate)(w263, w264) -> (w260:dbl[])
        n138 = call-poly <vilib>:"Plot Helper.vi"("error b percentage"=w265, "error a percentage"=w265, "y vector"=w266, "x vector"=w260) -> ("2D Plot Class Obj Array out"=→"2D Error Bar":refnum<class "2D Plot Datatype.lvclass">[])  [unwired: 2 in, 5 out]
      }
    }
  }
  n139 = for {
    tunnel: w23 -> [w292] mode=indexing
    tunnel: w22 -> [w291] mode=indexing
    tunnel: w21 -> [w290] mode=indexing
    tunnel: w20 -> [w289] mode=indexing
    tunnel: [w288] -> w18 mode=indexing
    tunnel: [w287] -> w17 mode=indexing
    tunnel: [w286] -> w16 mode=indexing
    tunnel: [w285] -> w15 mode=indexing
    tunnel: [w284] -> w14 mode=indexing
    tunnel: [w283] -> w13 mode=indexing
    tunnel: [w282] -> w12 mode=indexing
    tunnel: [w281] -> w11 mode=indexing
    tunnel: [w280] -> w10 mode=indexing
    tunnel: [w279] -> w9 mode=indexing
    tunnel: [w278] -> w8 mode=indexing
    tunnel: [w277] -> w7 mode=indexing
    n140 = Unbundle(w289) -> (w279:dbl, w278:dbl, w277:dbl)
    n141 = Unbundle(w291) -> ("sigma_A (Oe)"=w285:dbl, "sigma_A (Oe)"=w284:dbl, w283:dbl)
    n142 = Unbundle(w290) -> (w282:dbl, w281:dbl, w280:dbl)
    n143 = Unbundle(w292) -> ("intercept"=w288:dbl, "intercept"=w287:dbl, w286:dbl)
  }
  n144 = case shown="True" "Write to ITX" {
    tunnel: w19 -> [_ w308]
    tunnel: w18 -> [_ w307]
    tunnel: w17 -> [_ w306]
    tunnel: w16 -> [_ w305]
    tunnel: w15 -> [_ w304]
    tunnel: w14 -> [_ w303]
    tunnel: w13 -> [_ w302]
    tunnel: w12 -> [_ w301]
    tunnel: w11 -> [_ w300]
    tunnel: w10 -> [_ w299]
    tunnel: w9 -> [_ w298]
    tunnel: w8 -> [_ w297]
    tunnel: w7 -> [_ w296]
    tunnel: w6 -> [_ w295]
    tunnel: w5 -> [_ w294]
    frame False {
    }
    frame True {
      n145 = Build Cluster Array(w308, w307, w306, w305, w304, w303, w302, w301, w300, w299, w298, w297, w296, w295, w294) -> (w293:cluster{dbl[]}[])
      n146 = call <userlib>:"LV to ITX AutoPlot.vi"("filename"="filename", "path"="saved ITX", "Notes"="Comment", "Data"=w293, "wavenames (.Vx, etc)"=string[] ["Vsg", "Bc+", "Bc-", "Bc average", "Bc+ error", "Bc- error", "Bc error", "g+", "g-", "g average", "g+ error", "g- error", "g error average", "Coupling factor", "Coupling factor error"]) -> ()  [unwired: 10 in, 1 out]
    }
  }
